vi "transfer char run_subvi_7_25_12a_JW.vi"(0 "VISA session":refnum<visa-resource-name>="GPIB0::17::INSTR", 5 "Var1 sweep settings":T4={"start"=40.0, "stop"=-40.0, "step (linear only)"=-1.0, "sweep spacing (linear: 0)"=0, "sweep mode"=FALSE, "compliance (V)"=100.0, "compliance (A)"=0.001} {"compliance (A)" format="%^.2e"; "compliance (V)" format="%.2f"; "sweep spacing (linear: 0)" items=["linear", "log 10", "log 25", "log 50"]; "step (linear only)" format="%.2f"; "stop" format="%.2f"; "start" format="%.2f"}, 7 "Var2 step settings":T3={"compliance (A)"=0.001, "compliance (V)"=100.0, "start"=-2.0, "total points"=2, "step"=-38.0} {"step" format="%.2f"; "start" format="%.2f"; "compliance (V)" format="%.2f"; "compliance (A)" format="%^.2e"}, 9 "integration time":u32(slide) scale=0.0..2.0, 11 "Input Path":path, 13 "Sample Properties:":T1 {"Date Created" format="%<%x>T"}) -> (1 "Trap Density-STS":dbl, 3 "Trap Density-VT":dbl, 4 "Mobility":dbl, 6 "graphic display":cluster{"trace":dbl[], "trace":dbl[]}(graph), 8 "On/Off Current":dbl, 10 "XY Graph":cluster{dbl[], "trace":dbl[]}[](graph), 12 "Vt":dbl, 14 "STS":dbl, 15 "error?":errorcluster)   [LabVIEW 2011]
uses:
  <vilib>/Utility/file.llb/Write To Spreadsheet File (DBL).vi
  <vilib>/Utility/file.llb/Read From Spreadsheet File (string).vi
  <vilib>/Utility/file.llb/Write To Spreadsheet File (string).vi
  <vilib>/Analysis/NI_AALPro.lvlib
panel:
  out "Array":string[][](array[string])
  in  "Output Path":path
  in  "Temp (K)":dbl=0.001 format="%^.2e"
  in  "NumPts":dbl=5.0
  out "Numeric":dbl
  out "Max R":i32[](listbox)
  out "min r":dbl
  out "max r":dbl
  out "error? 2":errorcluster
  in  "MAXIMUM":ext format="%.2e"
  in  "MINIMUM":ext=-1e-05 format="%_2e"
  out "graphic display 2":cluster{"trace":dbl[], "trace":dbl[]}(graph)
  in  "Y1 axis":string="Id"
  in  "Y2 axis settings":T2 {"MAXIMUM" format="%.9f"; "MINIMUM" format="%.9f"}
  in  "wait time parameter":dbl=1.0
  in  "Value (Either V or A) 4":dbl
  in  "Value (Either V or A) 3":dbl
  in  "Value (Either V or A) 2":dbl
  in  "Value (V or A)":dbl
  in  "compliance (A)":dbl=0.001 format="%^.2e"
  in  "compliance (V)":dbl=100.0 format="%^.2e"
  in  "Iname":string="Is"
  in  "Vname":string="Vs"
  in  "Function":u16(ring)=4 items=["disabled", "Var1", "Var2", "Var1'", "Constant"]
  in  "Mode":u16(ring)=4 items=["V", "I", "VPulse", "IPulse", "Common"]
  in  "Iname 4":string="I4"
  in  "Vname 4":string="V4"
  in  "Function 4":u16(ring)=4 items=["disabled", "Var1", "Var2", "Var1'", "Constant"]
  in  "Mode 4":u16(ring) items=["V", "I", "VPulse", "IPulse", "Common"]
  in  "Iname 3":string="Ig"
  in  "Vname 3":string="Vg"
  in  "Function 3":u16(ring)=1 items=["disabled", "Var1", "Var2", "Var1'", "Constant"]
  in  "Mode 3":u16(ring) items=["V", "I", "VPulse", "IPulse", "Common"]
  in  "Iname 2":string="Id"
  in  "Vname 2":string="Vd"
  in  "Function 2":u16(ring)=2 items=["disabled", "Var1", "Var2", "Var1'", "Constant"]
  in  "Mode 2":u16(ring) items=["V", "I", "VPulse", "IPulse", "Common"]
  in  "reset":bool=TRUE
  # "SMU1"
  # "SMU2"
  # "SMU3"
  # "SMU4"
  # "Sample Properties:"
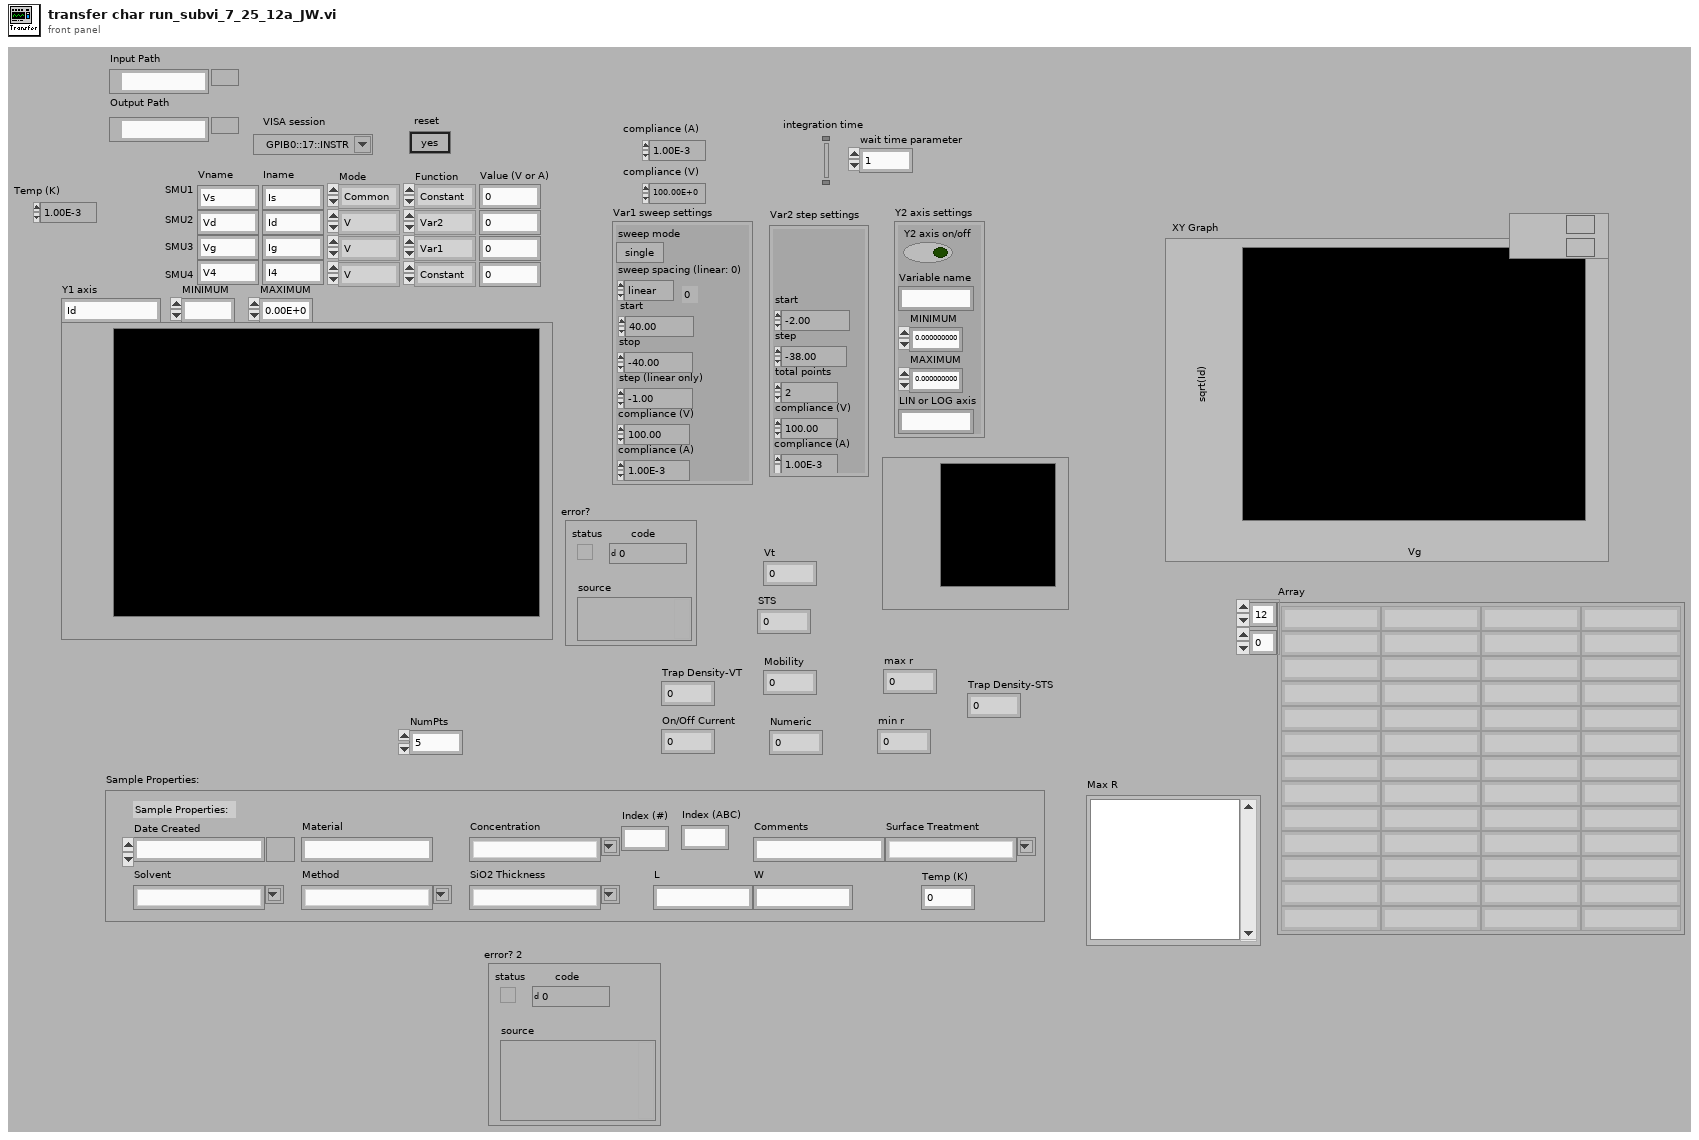
[diagram p1: front panel]
types:
  T1 = cluster{"Date Created":timestamp, "Material":string, "Solvent":string, "Concentration":string, "Method":string, "SiO2 Thickness":string, "Index (#)":string, "Index (ABC)":string, "L":string, "W":string, "Surface Treatment":string, "Comments":string, "Temp (K)":dbl}
  T2 = cluster{"Y2 axis on/off":bool, "MINIMUM":ext, "MAXIMUM":ext, "Variable name":string, "LIN or LOG axis":string}
  T3 = cluster{"compliance (A)":dbl, "compliance (V)":dbl, "start":dbl, "total points":u16, "step":dbl}
  T4 = cluster{"start":dbl, "stop":dbl, "step (linear only)":dbl, "sweep spacing (linear: 0)":u16, "sweep mode":bool, "compliance (V)":dbl, "compliance (A)":dbl}
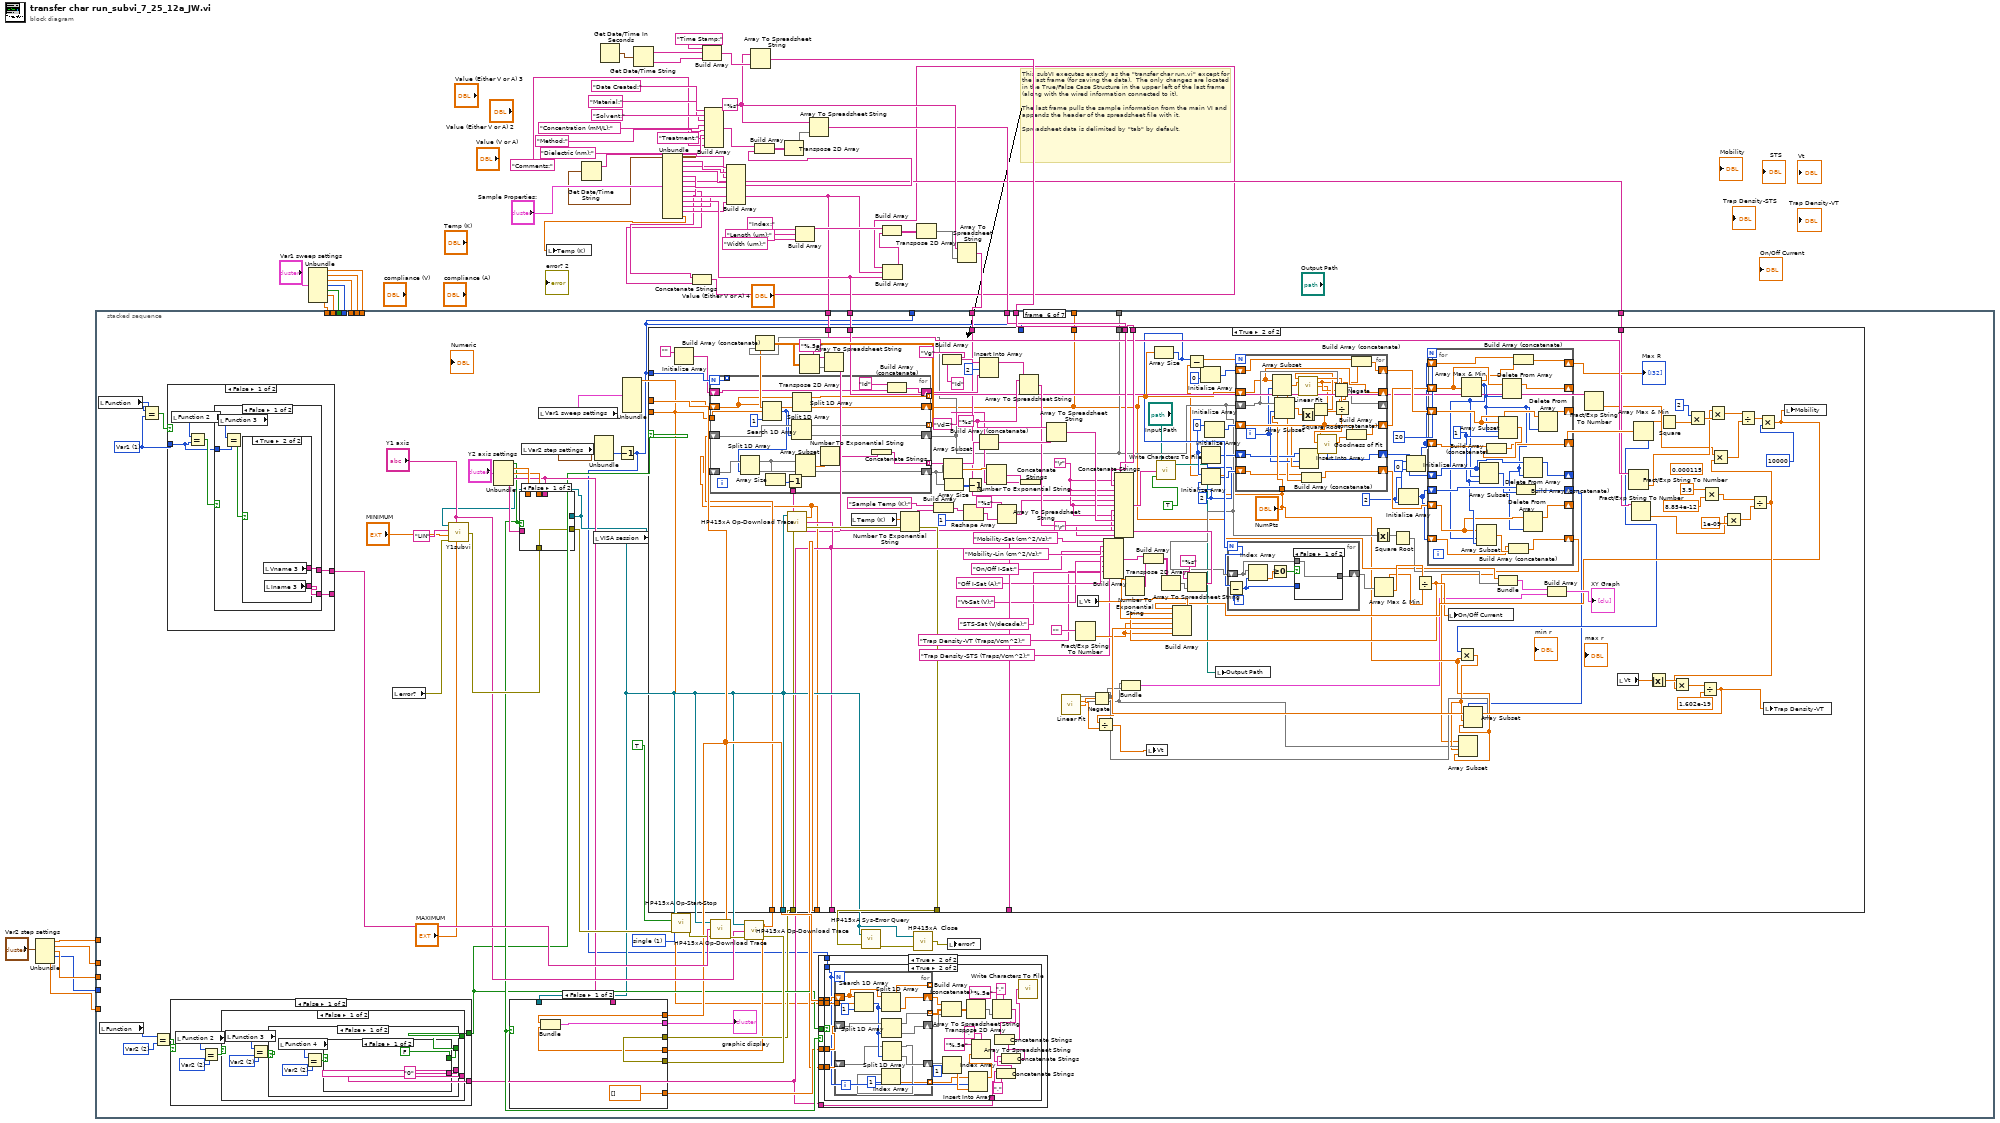
[diagram p0: block diagram]
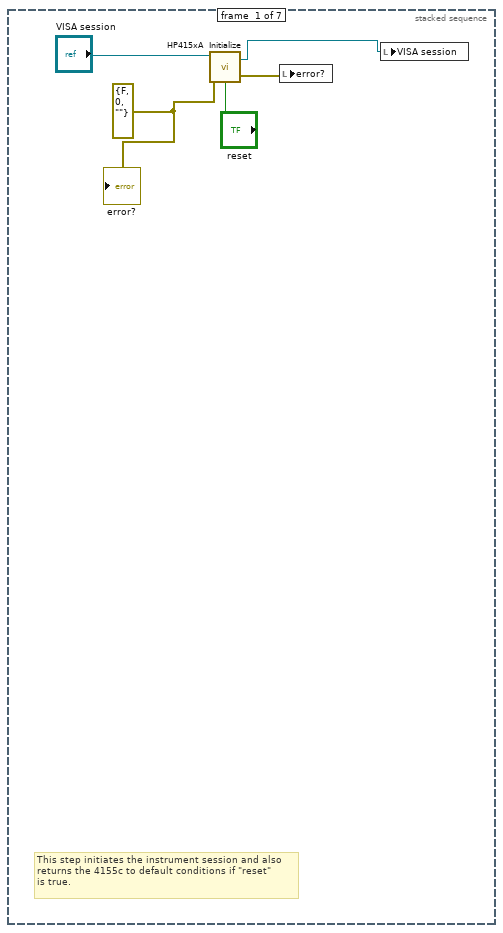
[diagram p2: hidden frame]
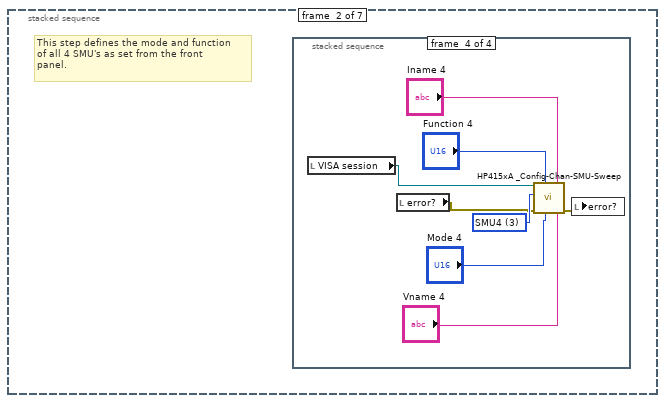
[diagram p3: hidden frame]
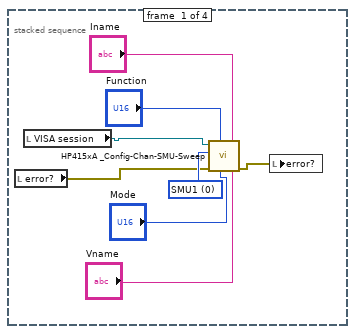
[diagram p4: hidden frame]
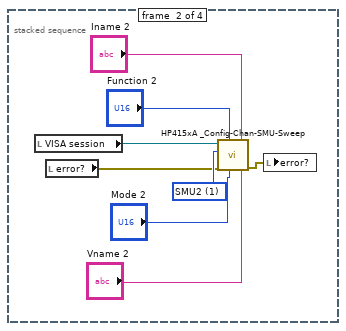
[diagram p5: hidden frame]
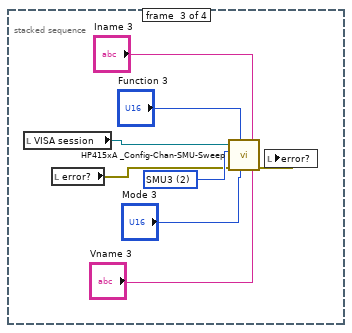
[diagram p6: hidden frame]
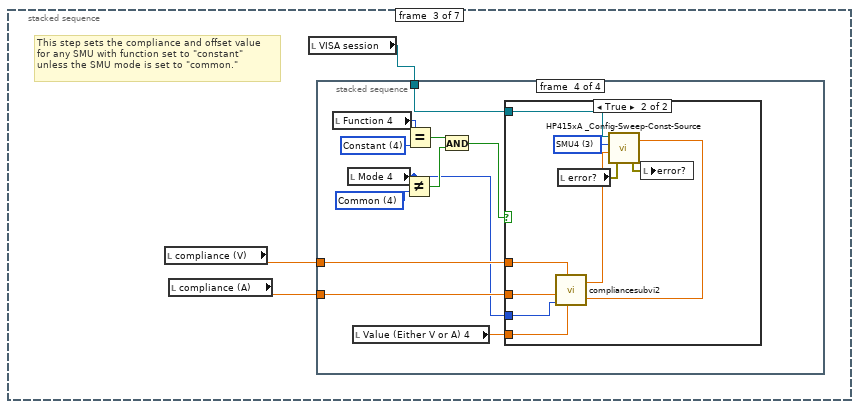
[diagram p7: hidden frame]
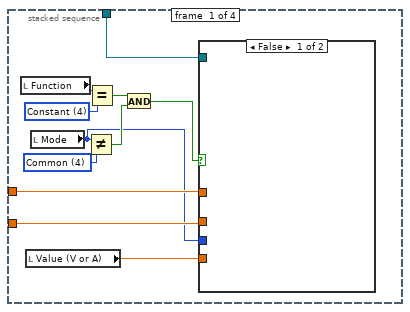
[diagram p8: hidden frame]
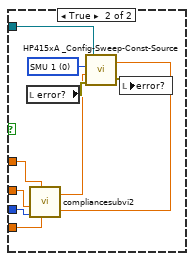
[diagram p9: hidden frame]
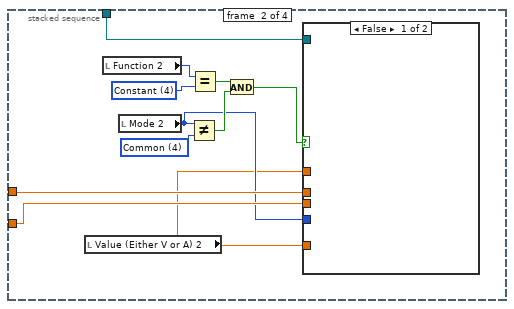
[diagram p10: hidden frame]
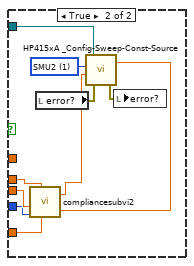
[diagram p11: hidden frame]
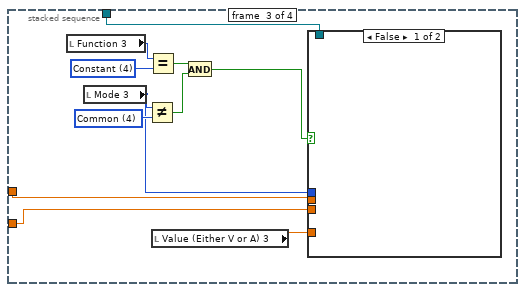
[diagram p12: hidden frame]
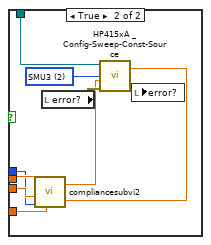
[diagram p13: hidden frame]
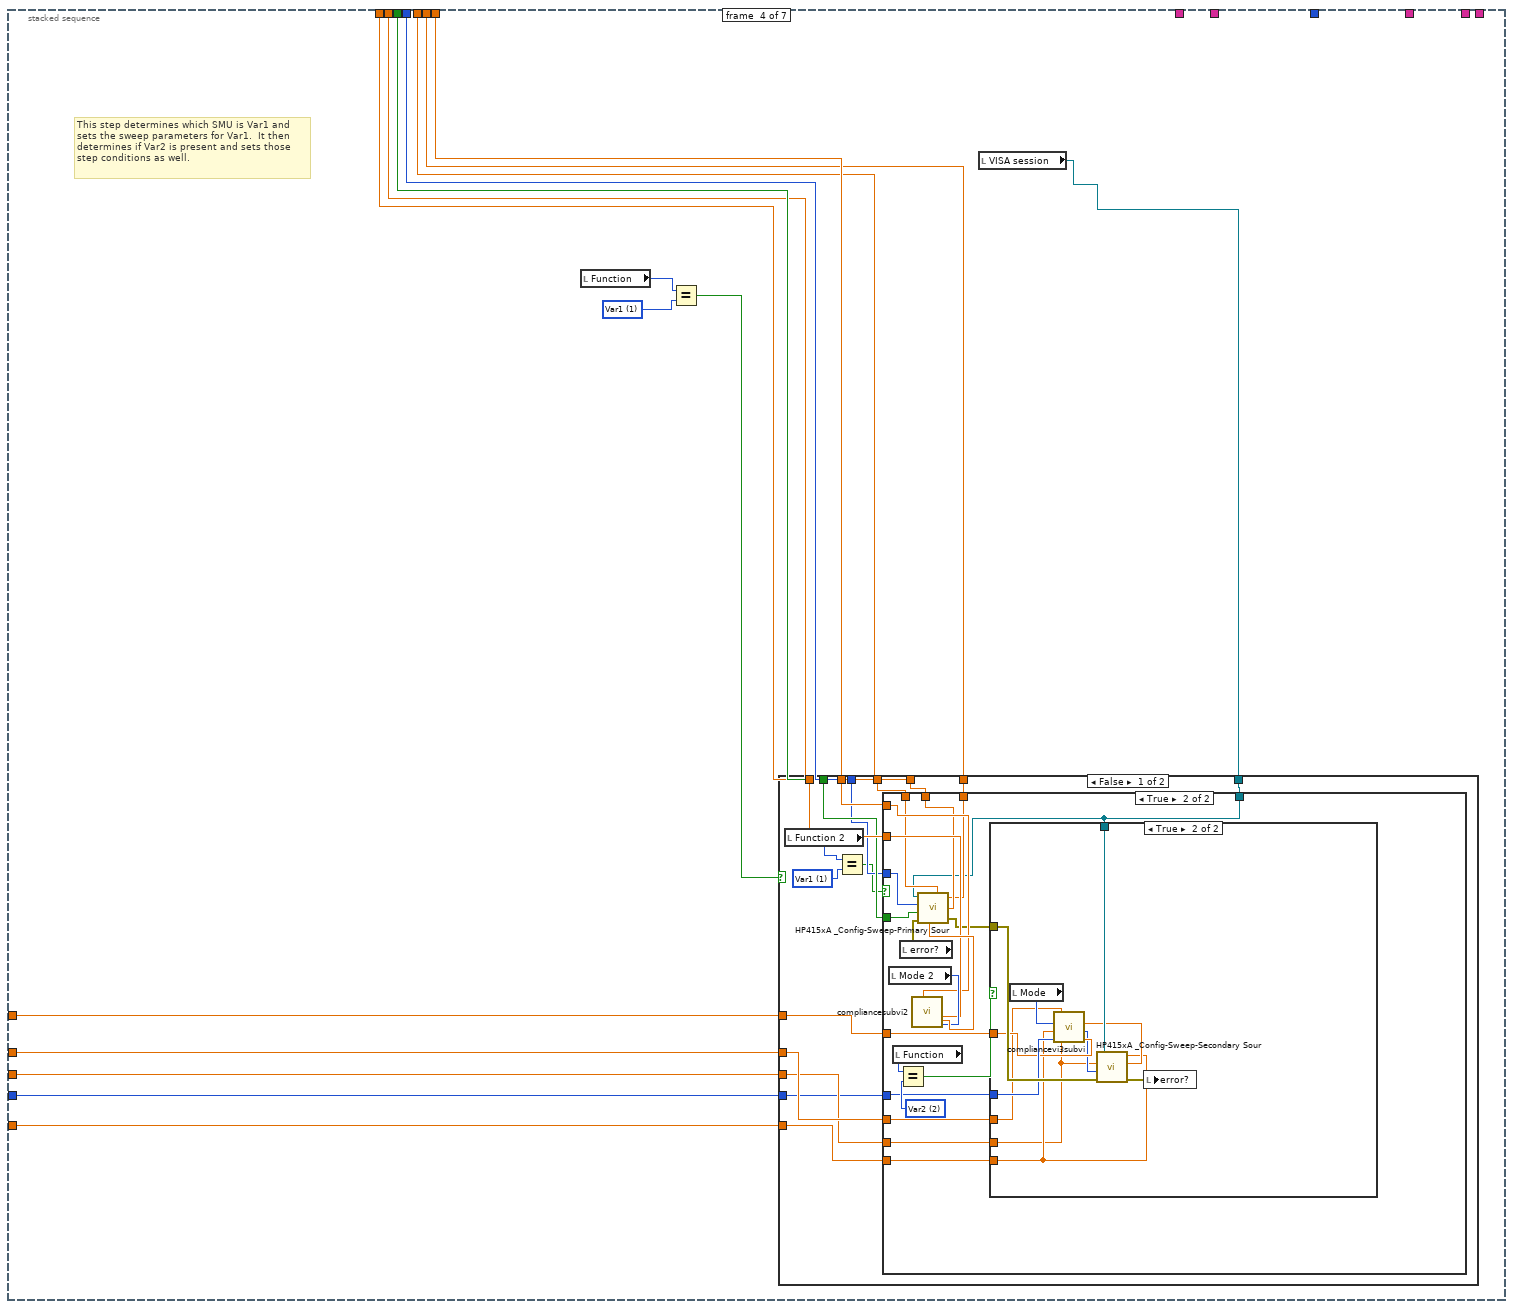
[diagram p15: hidden frame]
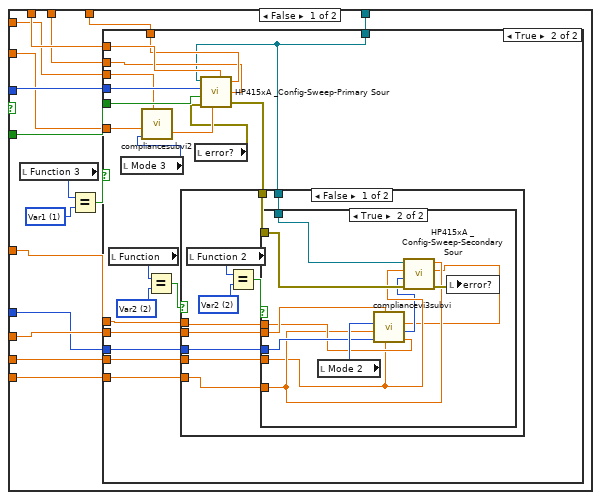
[diagram p16: hidden frame]
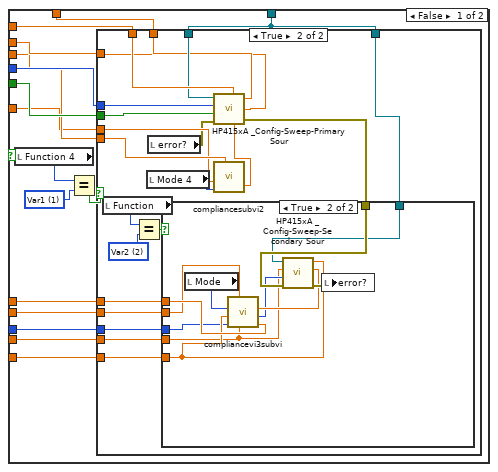
[diagram p17: hidden frame]
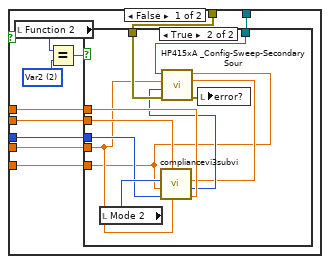
[diagram p19: hidden frame]
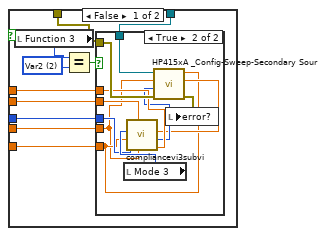
[diagram p20: hidden frame]
diagram:
  w31 = "%s"
  # "This subVI executes exactly as the \"transfer char run.vi\" except for the last frame (for saving the data).  The only changes are located in the True/False Case Structure in the upper left of the last frame (along with the wired information connected to it). \n\nThe last frame pulls the sample information from the main VI and appends the header of the spreadsheet file with it.\n\nSpreadsheet data is delimited by \"tab\" by default."
  n1 = Unbundle("Var2 step settings") -> ("compliance (A)"=w49:dbl, "compliance (V)"=w48:dbl, "start"=w47:dbl, "total points"=w46:u16, "step"=w45:dbl)
  n2 = Unbundle("Var1 sweep settings") -> ("start"=w57:dbl, "stop"=w56:dbl, "step (linear only)"=w55:dbl, "sweep spacing (linear: 0)"=w54:u16, "sweep mode"=w53:bool, "compliance (V)"=w52:dbl, "compliance (A)"=w51:dbl)
  n3 = Get Date/Time In Seconds() -> (seconds since 1Jan1904=w38:timestamp)
  n4 = Get Date/Time String(seconds (now)=w38) -> (date string=w37:string, time string=w36:string)  [unwired: 2 in]
  n5 = Unbundle("Sample Properties:") -> ("Date Created"=w16:timestamp, "Material"=w15:string, "Solvent"=w11:string, "Concentration"=w10:string, "Method"=w14:string, "SiO2 Thickness"=w9:string, "Index (#)"=w4:string, "Index (ABC)"=w3:string, "L"=w7:string, "W"=w8:string, "Surface Treatment"=w6:string, "Comments"=w5:string, "Temp (K)"=w1:dbl)
  n6 = local write "Temp (K)"(w1) -> ()
  n7 = Get Date/Time String(seconds (now)=w16) -> (date string=w43:string)  [unwired: 2 in, 1 out]
  n8 = Concatenate Strings(w4, w3) -> (w2:string)
  n9 = Build Array("Time Stamp:", w37, w36) -> (w35:string[])
  n10 = Build Array("Date Created:", "Material:", "Solvent:", "Concentration (mM/L):", "Method:", "Dielectric (nm):", "Treatment:", "Comments:") -> (w26:string[])
  n11 = Build Array(w43, w15, w11, w10, w14, w9, w6, w5) -> (w25:string[])
  n12 = Array To Spreadsheet String(array=w35, 3:w31) -> (spreadsheet string=w27:string)  [unwired: 1 in]
  n13 = Build Array(w26, w25) -> (w24:string[][])
  n14 = Transpose 2D Array(2D array=w24) -> (transposed array=w23:string[][])
  n15 = Build Array("Index:", "Length (um):", "Width (um):") -> (w22:string[])
  n16 = Array To Spreadsheet String(array=w23, 3:w31) -> (spreadsheet string=w30:string)  [unwired: 1 in]
  n17 = Build Array(w2, w7, w8) -> (w21:string[])
  n18 = Build Array(w22, w21) -> (w20:string[][])
  n19 = Transpose 2D Array(2D array=w20) -> (transposed array=w19:string[][])
  n20 = Array To Spreadsheet String(array=w19, 3:w31) -> (spreadsheet string=w18:string)  [unwired: 1 in]
  n21 = stacked-sequence {
    tunnel: w57 -> [_ _ _ w194 _ _ _]
    tunnel: w56 -> [_ _ _ w193 _ _ _]
    tunnel: w55 -> [_ _ _ w192 _ _ _]
    tunnel: w54 -> [_ _ _ w191 _ _ _]
    tunnel: w53 -> [_ _ _ w190 _ _ _]
    tunnel: w52 -> [_ _ _ w189 _ _ _]
    tunnel: w51 -> [_ _ _ w188 _ _ _]
    tunnel: w49 -> [_ _ _ w187 _ _ _]
    tunnel: w48 -> [_ _ _ w186 _ _ _]
    tunnel: w47 -> [_ _ _ w185 _ _ _]
    tunnel: w46 -> [_ _ _ w184 _ _ _]
    tunnel: w45 -> [_ _ _ w183 _ _ _]
    tunnel: w27 -> [_ _ _ _ _ w557 _]
    tunnel: w30 -> [_ _ _ _ _ w556 _]
    tunnel: w18 -> [_ _ _ _ _ w555 _]
    tunnel: [_ _ _ _ _ w554 _] -> _
    tunnel: [_ _ _ _ _ w553 _] -> _
    tunnel: [_ _ _ _ _ w550 _] -> _
    tunnel: w8 -> [_ _ _ _ _ w552 _]
    tunnel: w7 -> [_ _ _ _ _ w551 _]
    tunnel: w9 -> [_ _ _ _ _ w549 _]
    frame #0 {
      w62 = errorcluster {"status"=FALSE, "code"=0, "source"=""} ("error out")
      # "This step initiates the instrument session and also\nreturns the 4155c to default conditions if \"reset\"\nis true."
      n22 = call "HP415xA  Initialize.vi"("instrument descriptor"="VISA session", "reset"="reset", "error in (no error)"=w62) -> ("VISA session"=w59:refnum<visa-resource-name>, "error out"=w61:errorcluster)  [unwired: 2 in]
      n23 = local write "error?"(w61) -> ()
      n24 = local write "VISA session"(w59) -> ()
      "error?" <- w62
    }
    frame #1 {
      # "This step defines the mode and function\nof all 4 SMU's as set from the front\npanel."
      n25 = stacked-sequence {
        frame #0 {
          w71 = u32 0 items=["SMU1  ", "SMU2  ", "SMU3  ", "SMU4  ", "SMU5  ", "SMU6  "] ("unit to configure")
          n26 = local read "error?"() -> (w66:errorcluster)
          n27 = local read "VISA session"() -> (w64:refnum<visa-resource-name>)
          n28 = call "HP415xA _Config-Chan-SMU-Sweep.vi"("V name (max 6 chars)"="Vname", "I name (max 6 chars)"="Iname", "mode"="Mode", "function"="Function", "error in (no error)"=w66, "unit to configure"=w71, "VISA session"=w64) -> ("error out"=w65:errorcluster)  [unwired: 2 in]
          n29 = local write "error?"(w65) -> ()
        }
        frame #1 {
          w75 = u32 1 items=["SMU1  ", "SMU2  ", "SMU3  ", "SMU4  ", "SMU5  ", "SMU6  "] ("unit to configure")
          n30 = local read "VISA session"() -> (w72:refnum<visa-resource-name>)
          n31 = local read "error?"() -> (w73:errorcluster)
          n32 = call "HP415xA _Config-Chan-SMU-Sweep.vi"("V name (max 6 chars)"="Vname 2", "I name (max 6 chars)"="Iname 2", "mode"="Mode 2", "function"="Function 2", "error in (no error)"=w73, "unit to configure"=w75, "VISA session"=w72) -> ("error out"=w74:errorcluster)  [unwired: 2 in]
          n33 = local write "error?"(w74) -> ()
        }
        frame #2 {
          w83 = u32 2 items=["SMU1  ", "SMU2  ", "SMU3  ", "SMU4  ", "SMU5  ", "SMU6  "] ("unit to configure")
          n34 = local read "VISA session"() -> (w80:refnum<visa-resource-name>)
          n35 = local read "error?"() -> (w81:errorcluster)
          n36 = call "HP415xA _Config-Chan-SMU-Sweep.vi"("V name (max 6 chars)"="Vname 3", "I name (max 6 chars)"="Iname 3", "mode"="Mode 3", "function"="Function 3", "error in (no error)"=w81, "unit to configure"=w83, "VISA session"=w80) -> ("error out"=w82:errorcluster)  [unwired: 2 in]
          n37 = local write "error?"(w82) -> ()
        }
        frame #3 {
          w91 = u32 3 items=["SMU1  ", "SMU2  ", "SMU3  ", "SMU4  ", "SMU5  ", "SMU6  "] ("unit to configure")
          n38 = local read "VISA session"() -> (w88:refnum<visa-resource-name>)
          n39 = local read "error?"() -> (w90:errorcluster)
          n40 = call "HP415xA _Config-Chan-SMU-Sweep.vi"("V name (max 6 chars)"="Vname 4", "I name (max 6 chars)"="Iname 4", "mode"="Mode 4", "function"="Function 4", "error in (no error)"=w90, "unit to configure"=w91, "VISA session"=w88) -> ("error out"=w89:errorcluster)  [unwired: 2 in]
          n41 = local write "error?"(w89) -> ()
        }
      }
    }
    frame #2 {
      # "This step sets the compliance and offset value\nfor any SMU with function set to \"constant\"\nunless the SMU mode is set to \"common.\""
      n42 = local read "compliance (V)"() -> (w97:dbl)
      n43 = local read "compliance (A)"() -> (w98:dbl)
      n44 = local read "VISA session"() -> (w96:refnum<visa-resource-name>)
      n45 = stacked-sequence {
        tunnel: w96 -> [w107 w127 w146 w166]
        tunnel: w98 -> [w101 w123 w144 w164]
        tunnel: w97 -> [w100 w122 w143 w165]
        frame #0 {
          w105 = u16 4 items=["V", "I", "VPulse", "IPulse", "Common"] ("Mode")
          w109 = u16 4 items=["disabled", "Var1", "Var2", "Var1'", "Constant"] ("Function")
          n46 = local read "Function"() -> (w108:u16)
          n47 = local read "Value (V or A)"() -> (w102:dbl)
          n48 = local read "Mode"() -> (w99:u16)
          n49 = Not Equal?(x=w99, y=w105) -> (x != y?=w104:bool)
          n50 = Equal?(x=w108, y=w109) -> (x = y?=w106:bool)
          n51 = And(x=w106, y=w104) -> (x .and. y?=w103:bool)
          n52 = case shown="False" w103 {
            tunnel: w107 -> [_ w119]
            tunnel: w100 -> [_ w115]
            tunnel: w101 -> [_ w114]
            tunnel: w102 -> [_ w111]
            tunnel: w99 -> [_ w112]
            frame False {
            }
            frame True {
              w118 = u16 0 items=["SMU 1", "SMU2", "SMU3", "SMU4", "SMU5", "SMU6", "VSU1", "VSU2"] ("unit (SMU1:0)")
              n53 = local read "error?"() -> (w117:errorcluster)
              n54 = call "compliancesubvi2.vi"("Value1"=w111, "compliance (V)"=w115, "Mode"=w112, "compliance (A)"=w114) -> ("compliance"=w113:dbl, "constant"=w110:dbl)  [unwired: 2 in]
              n55 = call "HP415xA _Config-Sweep-Const-Source.vi"("compliance (SMUs only)"=w113, "error in (no error)"=w117, "source (V or A)"=w110, "unit (SMU1:0)"=w118, "VISA session"=w119) -> ("error out"=w116:errorcluster)
              n56 = local write "error?"(w116) -> ()
            }
          }
        }
        frame #1 {
          w124 = u16 4 items=["V", "I", "VPulse", "IPulse", "Common"] ("Mode 2")
          w125 = u16 4 items=["disabled", "Var1", "Var2", "Var1'", "Constant"] ("Function 2")
          n57 = local read "Value (Either V or A) 2"() -> (w120:dbl)
          n58 = local read "Function 2"() -> (w126:u16)
          n59 = local read "Mode 2"() -> (w121:u16)
          n60 = Not Equal?(x=w121, y=w124) -> (x != y?=w129:bool)
          n61 = Equal?(x=w126, y=w125) -> (x = y?=w130:bool)
          n62 = And(x=w130, y=w129) -> (x .and. y?=w128:bool)
          n63 = case shown="False" w128 {
            tunnel: w127 -> [_ w140]
            tunnel: w122 -> [_ w138]
            tunnel: w123 -> [_ w137]
            tunnel: w120 -> [_ _]
            tunnel: w121 -> [_ w133]
            tunnel: w120 -> [_ w132]
            frame False {
            }
            frame True {
              w139 = u16 1 items=["SMU 1", "SMU2", "SMU3", "SMU4", "SMU5", "SMU6", "VSU1", "VSU2"] ("unit (SMU1:0)")
              n64 = call "compliancesubvi2.vi"("Value1"=w132, "compliance (V)"=w138, "Mode"=w133, "compliance (A)"=w137) -> ("compliance"=w136:dbl, "constant"=w131:dbl)  [unwired: 2 in]
              n65 = local read "error?"() -> (w135:errorcluster)
              n66 = call "HP415xA _Config-Sweep-Const-Source.vi"("compliance (SMUs only)"=w136, "error in (no error)"=w135, "source (V or A)"=w131, "unit (SMU1:0)"=w139, "VISA session"=w140) -> ("error out"=w134:errorcluster)
              n67 = local write "error?"(w134) -> ()
            }
          }
        }
        frame #2 {
          w148 = u16 4 items=["V", "I", "VPulse", "IPulse", "Common"] ("Mode 2")
          w149 = u16 4 items=["disabled", "Var1", "Var2", "Var1'", "Constant"] ("Function 2")
          n68 = local read "Function 3"() -> (w147:u16)
          n69 = local read "Mode 3"() -> (w142:u16)
          n70 = Not Equal?(x=w142, y=w148) -> (x != y?=w150:bool)
          n71 = Equal?(x=w147, y=w149) -> (x = y?=w151:bool)
          n72 = local read "Value (Either V or A) 3"() -> (w145:dbl)
          n73 = And(x=w151, y=w150) -> (x .and. y?=w141:bool)
          n74 = case shown="False" w141 {
            tunnel: w146 -> [_ w159]
            tunnel: w145 -> [_ w153]
            tunnel: w144 -> [_ w156]
            tunnel: w143 -> [_ w155]
            tunnel: w142 -> [_ w154]
            frame False {
            }
            frame True {
              w158 = u16 2 items=["SMU 1", "SMU2", "SMU3", "SMU4", "SMU5", "SMU6", "VSU1", "VSU2"] ("unit (SMU1:0)")
              n75 = call "compliancesubvi2.vi"("Value1"=w153, "compliance (V)"=w155, "Mode"=w154, "compliance (A)"=w156) -> ("compliance"=w157:dbl, "constant"=w152:dbl)  [unwired: 2 in]
              n76 = local read "error?"() -> (w161:errorcluster)
              n77 = call "HP415xA _Config-Sweep-Const-Source.vi"("compliance (SMUs only)"=w157, "error in (no error)"=w161, "source (V or A)"=w152, "unit (SMU1:0)"=w158, "VISA session"=w159) -> ("error out"=w160:errorcluster)
              n78 = local write "error?"(w160) -> ()
            }
          }
        }
        frame #3 {
          w168 = u16 4 items=["V", "I", "VPulse", "IPulse", "Common"] ("Mode 4")
          w169 = u16 4 items=["disabled", "Var1", "Var2", "Var1'", "Constant"] ("Function 4")
          n79 = local read "Function 4"() -> (w170:u16)
          n80 = local read "Mode 4"() -> (w163:u16)
          n81 = local read "Value (Either V or A) 4"() -> (w162:dbl)
          n82 = Not Equal?(x=w163, y=w168) -> (x != y?=w171:bool)
          n83 = Equal?(x=w170, y=w169) -> (x = y?=w172:bool)
          n84 = And(x=w172, y=w171) -> (x .and. y?=w167:bool)
          n85 = case shown="True" w167 {
            tunnel: w166 -> [_ w181]
            tunnel: w165 -> [_ w177]
            tunnel: w164 -> [_ w178]
            tunnel: w163 -> [_ w176]
            tunnel: w162 -> [_ w175]
            frame False {
            }
            frame True {
              w182 = u16 3 items=["SMU 1", "SMU2", "SMU3", "SMU4", "SMU5", "SMU6", "VSU1", "VSU2"] ("unit (SMU1:0)")
              n86 = call "compliancesubvi2.vi"("Value1"=w175, "compliance (V)"=w177, "Mode"=w176, "compliance (A)"=w178) -> ("compliance"=w174:dbl, "constant"=w173:dbl)  [unwired: 2 in]
              n87 = local read "error?"() -> (w180:errorcluster)
              n88 = call "HP415xA _Config-Sweep-Const-Source.vi"("compliance (SMUs only)"=w174, "error in (no error)"=w180, "source (V or A)"=w173, "unit (SMU1:0)"=w182, "VISA session"=w181) -> ("error out"=w179:errorcluster)
              n89 = local write "error?"(w179) -> ()
            }
          }
        }
      }
    }
    frame #3 {
      w198 = u16 1 items=["disabled", "Var1", "Var2", "Var1'", "Constant"] ("Function")
      # "This step determines which SMU is Var1 and\nsets the sweep parameters for Var1.  It then\ndetermines if Var2 is present and sets those\nstep conditions as well."
      n90 = local read "Function"() -> (w197:u16)
      n91 = Equal?(x=w197, y=w198) -> (x = y?=w196:bool)
      n92 = local read "VISA session"() -> (w195:refnum<visa-resource-name>)
      n93 = case shown="False" w196 {
        tunnel: w189 -> [w211 w487]
        tunnel: w188 -> [w212 w486]
        tunnel: w191 -> [w209 w485]
        tunnel: w190 -> [w210 w484]
        tunnel: w192 -> [w206 w483]
        tunnel: w193 -> [w205 w482]
        tunnel: w194 -> [w207 w481]
        tunnel: w195 -> [w208 w470]
        tunnel: w187 -> [w203 w476]
        tunnel: w186 -> [w202 w475]
        tunnel: w185 -> [w201 w474]
        tunnel: w184 -> [w200 w473]
        tunnel: w183 -> [w199 w472]
        frame False {
          w214 = u16 1 items=["disabled", "Var1", "Var2", "Var1'", "Constant"] ("Function")
          n94 = local read "Function 2"() -> (w213:u16)
          n95 = Equal?(x=w213, y=w214) -> (x = y?=w204:bool)
          n96 = case shown="True" w204 {
            tunnel: w212 -> [w220 w413]
            tunnel: w211 -> [w221 w412]
            tunnel: w210 -> [w222 w411]
            tunnel: w209 -> [w223 w410]
            tunnel: w208 -> [w227 w399]
            tunnel: w207 -> [w226 w409]
            tunnel: w206 -> [w224 w408]
            tunnel: w205 -> [w225 w407]
            tunnel: w203 -> [w219 w402]
            tunnel: w202 -> [w218 w401]
            tunnel: w201 -> [w216 w400]
            tunnel: w200 -> [w217 w397]
            tunnel: w199 -> [w215 w396]
            frame False {
              w230 = u16 1 items=["disabled", "Var1", "Var2", "Var1'", "Constant"] ("Function")
              n97 = local read "Function 3"() -> (w229:u16)
              n98 = Equal?(x=w229, y=w230) -> (x = y?=w228:bool)
              n99 = case shown="True" w228 {
                tunnel: w227 -> [w231 w324]
                tunnel: w226 -> [w243 w341]
                tunnel: w225 -> [w240 w340]
                tunnel: w224 -> [w239 w339]
                tunnel: w223 -> [w242 w338]
                tunnel: w222 -> [w241 w337]
                tunnel: w221 -> [w238 w336]
                tunnel: w220 -> [w237 w335]
                tunnel: w219 -> [w236 w328]
                tunnel: w218 -> [w235 w327]
                tunnel: w217 -> [w234 w326]
                tunnel: w216 -> [w233 w323]
                tunnel: w215 -> [w232 w322]
                frame False {
                  w246 = u16 1 items=["disabled", "Var1", "Var2", "Var1'", "Constant"] ("Function")
                  n100 = local read "Function 4"() -> (w245:u16)
                  n101 = Equal?(x=w245, y=w246) -> (x = y?=w244:bool)
                  n102 = case shown="True" w244 {
                    tunnel: w243 -> [_ w265]
                    tunnel: w231 -> [_ w264]
                    tunnel: w242 -> [_ w263]
                    tunnel: w241 -> [_ w262]
                    tunnel: w240 -> [_ w261]
                    tunnel: w239 -> [_ w260]
                    tunnel: w238 -> [_ w259]
                    tunnel: w237 -> [_ w258]
                    tunnel: w236 -> [_ w253]
                    tunnel: w235 -> [_ w252]
                    tunnel: w234 -> [_ w251]
                    tunnel: w233 -> [_ w250]
                    tunnel: w232 -> [_ w249]
                    tunnel: w231 -> [_ w247]
                    frame False {
                    }
                    frame True {
                      w256 = u16 2 items=["disabled", "Var1", "Var2", "Var1'", "Constant"] ("Function")
                      n103 = local read "Function"() -> (w255:u16)
                      n104 = Equal?(x=w255, y=w256) -> (x = y?=w254:bool)
                      n105 = local read "Mode 4"() -> (w267:u16)
                      n106 = local read "error?"() -> (w257:errorcluster)
                      n107 = call "compliancesubvi2.vi"("compliance (V)"=w259, "Mode"=w267, "compliance (A)"=w258) -> ("compliance"=w266:dbl)  [unwired: 3 in, 1 out]
                      n108 = call "HP415xA _Config-Sweep-Primary Sour.vi"("step (linear only)"=w260, "stop"=w261, "start"=w265, "compliance"=w266, "error in (no error)"=w257, "sweep mode"=w262, "sweep spacing (linear: 0)"=w263, "VISA session"=w264) -> ("error out"=w248:errorcluster)  [unwired: 2 in]
                      n109 = case shown="True" w254 {
                        tunnel: w253 -> [w274 w317]
                        tunnel: w252 -> [w273 w312]
                        tunnel: w251 -> [w272 w311]
                        tunnel: w250 -> [w271 w313]
                        tunnel: w249 -> [w270 w316]
                        tunnel: w248 -> [w269 w319]
                        tunnel: w247 -> [w268 w318]
                        frame False {
                          w277 = u16 2 items=["disabled", "Var1", "Var2", "Var1'", "Constant"] ("Function")
                          n110 = local read "Function 2"() -> (w276:u16)
                          n111 = Equal?(x=w276, y=w277) -> (x = y?=w275:bool)
                          n112 = case shown="True" w275 {
                            tunnel: w274 -> [w285 w305]
                            tunnel: w273 -> [w284 w306]
                            tunnel: w272 -> [w283 w304]
                            tunnel: w271 -> [w282 w302]
                            tunnel: w270 -> [w281 w300]
                            tunnel: w269 -> [w280 w310]
                            tunnel: w268 -> [w278 w309]
                            frame False {
                              w287 = u16 2 items=["disabled", "Var1", "Var2", "Var1'", "Constant"] ("Function")
                              n113 = local read "Function 3"() -> (w279:u16)
                              n114 = Equal?(x=w279, y=w287) -> (x = y?=w286:bool)
                              n115 = case shown="True" w286 {
                                tunnel: w285 -> [_ w293]
                                tunnel: w284 -> [_ w294]
                                tunnel: w283 -> [_ w295]
                                tunnel: w282 -> [_ w289]
                                tunnel: w281 -> [_ w290]
                                tunnel: w280 -> [w288 w299]
                                tunnel: w278 -> [_ w298]
                                frame False {
                                n116 = local write "error?"(w288) -> ()
                                }
                                frame True {
                                n117 = local read "Mode 3"() -> (w297:u16)
                                n118 = call "compliancevi3subvi.vi"("compliance (A)"=w293, "start"=w289, "compliance (V)"=w294, "total points"=w295, "step"=w290, "Mode"=w297) -> ("total points 2"=w292:u16, "compliance"=w291:dbl)  [unwired: 1 in, 1 out]
                                n119 = call "HP415xA _Config-Sweep-Secondary Sour.vi"("compliance"=w291, "step"=w290, "error in (no error)"=w299, "total points"=w292, "start"=w289, "VISA session"=w298) -> ("error out"=w296:errorcluster)  [unwired: 1 in]
                                n120 = local write "error?"(w296) -> ()
                                }
                              }
                            }
                            frame True {
                              n121 = local read "Mode 2"() -> (w308:u16)
                              n122 = call "compliancevi3subvi.vi"("compliance (A)"=w305, "start"=w302, "compliance (V)"=w306, "total points"=w304, "step"=w300, "Mode"=w308) -> ("total points 2"=w303:u16, "compliance"=w301:dbl)  [unwired: 1 in, 1 out]
                              n123 = call "HP415xA _Config-Sweep-Secondary Sour.vi"("compliance"=w301, "step"=w300, "error in (no error)"=w310, "total points"=w303, "start"=w302, "VISA session"=w309) -> ("error out"=w307:errorcluster)  [unwired: 1 in]
                              n124 = local write "error?"(w307) -> ()
                            }
                          }
                        }
                        frame True {
                          n125 = local read "Mode"() -> (w321:u16)
                          n126 = call "compliancevi3subvi.vi"("compliance (A)"=w317, "start"=w313, "compliance (V)"=w312, "total points"=w311, "step"=w316, "Mode"=w321) -> ("total points 2"=w314:u16, "compliance"=w315:dbl)  [unwired: 1 in, 1 out]
                          n127 = call "HP415xA _Config-Sweep-Secondary Sour.vi"("compliance"=w315, "step"=w316, "error in (no error)"=w319, "total points"=w314, "start"=w313, "VISA session"=w318) -> ("error out"=w320:errorcluster)  [unwired: 1 in]
                          n128 = local write "error?"(w320) -> ()
                        }
                      }
                    }
                  }
                }
                frame True {
                  w331 = u16 2 items=["disabled", "Var1", "Var2", "Var1'", "Constant"] ("Function")
                  n129 = local read "Function"() -> (w330:u16)
                  n130 = local read "Mode 3"() -> (w333:u16)
                  n131 = call "compliancesubvi2.vi"("compliance (V)"=w336, "Mode"=w333, "compliance (A)"=w335) -> ("compliance"=w334:dbl)  [unwired: 3 in, 1 out]
                  n132 = Equal?(x=w330, y=w331) -> (x = y?=w329:bool)
                  n133 = local read "error?"() -> (w332:errorcluster)
                  n134 = call "HP415xA _Config-Sweep-Primary Sour.vi"("step (linear only)"=w339, "stop"=w340, "start"=w341, "compliance"=w334, "error in (no error)"=w332, "sweep mode"=w337, "sweep spacing (linear: 0)"=w338, "VISA session"=w324) -> ("error out"=w325:errorcluster)  [unwired: 2 in]
                  n135 = case shown="False" w329 {
                    tunnel: w328 -> [w346 w391]
                    tunnel: w327 -> [w345 w390]
                    tunnel: w326 -> [w343 w389]
                    tunnel: w325 -> [w348 w394]
                    tunnel: w324 -> [w347 w393]
                    tunnel: w323 -> [w342 w386]
                    tunnel: w322 -> [w344 w385]
                    frame False {
                      w351 = u16 2 items=["disabled", "Var1", "Var2", "Var1'", "Constant"] ("Function")
                      n136 = local read "Function 2"() -> (w350:u16)
                      n137 = Equal?(x=w350, y=w351) -> (x = y?=w349:bool)
                      n138 = case shown="True" w349 {
                        tunnel: w348 -> [w358 w383]
                        tunnel: w347 -> [w357 w382]
                        tunnel: w346 -> [w356 w378]
                        tunnel: w345 -> [w355 w379]
                        tunnel: w344 -> [w352 w377]
                        tunnel: w343 -> [w354 w380]
                        tunnel: w342 -> [w353 w376]
                        frame False {
                          w361 = u16 2 items=["disabled", "Var1", "Var2", "Var1'", "Constant"] ("Function")
                          n139 = local read "Function 4"() -> (w360:u16)
                          n140 = Equal?(x=w360, y=w361) -> (x = y?=w359:bool)
                          n141 = case shown="True" w359 {
                            tunnel: w358 -> [w362 w371]
                            tunnel: w357 -> [_ w372]
                            tunnel: w356 -> [_ w368]
                            tunnel: w355 -> [_ w369]
                            tunnel: w354 -> [_ w367]
                            tunnel: w353 -> [_ w364]
                            tunnel: w352 -> [_ w363]
                            frame False {
                              n142 = local write "error?"(w362) -> ()
                            }
                            frame True {
                              n143 = local read "Mode 4"() -> (w373:u16)
                              n144 = call "compliancevi3subvi.vi"("compliance (A)"=w368, "start"=w364, "compliance (V)"=w369, "total points"=w367, "step"=w363, "Mode"=w373) -> ("total points 2"=w366:u16, "compliance"=w365:dbl)  [unwired: 1 in, 1 out]
                              n145 = call "HP415xA _Config-Sweep-Secondary Sour.vi"("compliance"=w365, "step"=w363, "error in (no error)"=w371, "total points"=w366, "start"=w364, "VISA session"=w372) -> ("error out"=w370:errorcluster)  [unwired: 1 in]
                              n146 = local write "error?"(w370) -> ()
                            }
                          }
                        }
                        frame True {
                          n147 = local read "Mode 2"() -> (w384:u16)
                          n148 = call "compliancevi3subvi.vi"("compliance (A)"=w378, "start"=w376, "compliance (V)"=w379, "total points"=w380, "step"=w377, "Mode"=w384) -> ("total points 2"=w375:u16, "compliance"=w374:dbl)  [unwired: 1 in, 1 out]
                          n149 = call "HP415xA _Config-Sweep-Secondary Sour.vi"("compliance"=w374, "step"=w377, "error in (no error)"=w383, "total points"=w375, "start"=w376, "VISA session"=w382) -> ("error out"=w381:errorcluster)  [unwired: 1 in]
                          n150 = local write "error?"(w381) -> ()
                        }
                      }
                    }
                    frame True {
                      n151 = local read "Mode"() -> (w395:u16)
                      n152 = call "compliancevi3subvi.vi"("compliance (A)"=w391, "start"=w386, "compliance (V)"=w390, "total points"=w389, "step"=w385, "Mode"=w395) -> ("total points 2"=w388:u16, "compliance"=w387:dbl)  [unwired: 1 in, 1 out]
                      n153 = call "HP415xA _Config-Sweep-Secondary Sour.vi"("compliance"=w387, "step"=w385, "error in (no error)"=w394, "total points"=w388, "start"=w386, "VISA session"=w393) -> ("error out"=w392:errorcluster)  [unwired: 1 in]
                      n154 = local write "error?"(w392) -> ()
                    }
                  }
                }
              }
            }
            frame True {
              w405 = u16 2 items=["disabled", "Var1", "Var2", "Var1'", "Constant"] ("Function")
              n155 = local read "Mode 2"() -> (w414:u16)
              n156 = local read "Function"() -> (w404:u16)
              n157 = Equal?(x=w404, y=w405) -> (x = y?=w403:bool)
              n158 = local read "error?"() -> (w406:errorcluster)
              n159 = call "compliancesubvi2.vi"("compliance (V)"=w412, "Mode"=w414, "compliance (A)"=w413) -> ("compliance"=w415:dbl)  [unwired: 3 in, 1 out]
              n160 = call "HP415xA _Config-Sweep-Primary Sour.vi"("step (linear only)"=w408, "stop"=w407, "start"=w409, "compliance"=w415, "error in (no error)"=w406, "sweep mode"=w411, "sweep spacing (linear: 0)"=w410, "VISA session"=w399) -> ("error out"=w398:errorcluster)  [unwired: 2 in]
              n161 = case shown="True" w403 {
                tunnel: w402 -> [w421 w464]
                tunnel: w401 -> [w420 w463]
                tunnel: w400 -> [w418 w459]
                tunnel: w399 -> [w423 w469]
                tunnel: w398 -> [w417 w468]
                tunnel: w397 -> [w419 w465]
                tunnel: w396 -> [w416 w461]
                frame False {
                  w425 = u16 2 items=["disabled", "Var1", "Var2", "Var1'", "Constant"] ("Function")
                  n162 = local read "Function 3"() -> (w424:u16)
                  n163 = Equal?(x=w424, y=w425) -> (x = y?=w422:bool)
                  n164 = case shown="True" w422 {
                    tunnel: w423 -> [w431 w457]
                    tunnel: w421 -> [w430 w454]
                    tunnel: w420 -> [w428 w452]
                    tunnel: w419 -> [w429 w453]
                    tunnel: w418 -> [w426 w450]
                    tunnel: w417 -> [w432 w456]
                    tunnel: w416 -> [w427 w448]
                    frame False {
                      w435 = u16 2 items=["disabled", "Var1", "Var2", "Var1'", "Constant"] ("Function")
                      n165 = local read "Function 4"() -> (w434:u16)
                      n166 = Equal?(x=w434, y=w435) -> (x = y?=w433:bool)
                      n167 = case shown="True" w433 {
                        tunnel: w432 -> [w436 w447]
                        tunnel: w431 -> [_ w446]
                        tunnel: w430 -> [_ w443]
                        tunnel: w429 -> [_ w444]
                        tunnel: w428 -> [_ w442]
                        tunnel: w427 -> [_ w438]
                        tunnel: w426 -> [_ w439]
                        frame False {
                          n168 = local write "error?"(w436) -> ()
                        }
                        frame True {
                          n169 = local read "Mode 4"() -> (w441:u16)
                          n170 = call "compliancevi3subvi.vi"("compliance (A)"=w443, "start"=w439, "compliance (V)"=w442, "total points"=w444, "step"=w438, "Mode"=w441) -> ("total points 2"=w440:u16, "compliance"=w437:dbl)  [unwired: 1 in, 1 out]
                          n171 = call "HP415xA _Config-Sweep-Secondary Sour.vi"("compliance"=w437, "step"=w438, "error in (no error)"=w447, "total points"=w440, "start"=w439, "VISA session"=w446) -> ("error out"=w445:errorcluster)  [unwired: 1 in]
                          n172 = local write "error?"(w445) -> ()
                        }
                      }
                    }
                    frame True {
                      n173 = local read "Mode 3"() -> (w458:u16)
                      n174 = call "compliancevi3subvi.vi"("compliance (A)"=w454, "start"=w450, "compliance (V)"=w452, "total points"=w453, "step"=w448, "Mode"=w458) -> ("total points 2"=w451:u16, "compliance"=w449:dbl)  [unwired: 1 in, 1 out]
                      n175 = call "HP415xA _Config-Sweep-Secondary Sour.vi"("compliance"=w449, "step"=w448, "error in (no error)"=w456, "total points"=w451, "start"=w450, "VISA session"=w457) -> ("error out"=w455:errorcluster)  [unwired: 1 in]
                      n176 = local write "error?"(w455) -> ()
                    }
                  }
                }
                frame True {
                  n177 = local read "Mode"() -> (w466:u16)
                  n178 = call "compliancevi3subvi.vi"("compliance (A)"=w464, "start"=w459, "compliance (V)"=w463, "total points"=w465, "step"=w461, "Mode"=w466) -> ("total points 2"=w460:u16, "compliance"=w462:dbl)  [unwired: 1 in, 1 out]
                  n179 = call "HP415xA _Config-Sweep-Secondary Sour.vi"("compliance"=w462, "step"=w461, "error in (no error)"=w468, "total points"=w460, "start"=w459, "VISA session"=w469) -> ("error out"=w467:errorcluster)  [unwired: 1 in]
                  n180 = local write "error?"(w467) -> ()
                }
              }
            }
          }
        }
        frame True {
          w478 = u16 2 items=["disabled", "Var1", "Var2", "Var1'", "Constant"] ("Function 2")
          n181 = local read "error?"() -> (w480:errorcluster)
          n182 = local read "Mode"() -> (w488:u16)
          n183 = local read "Function 2"() -> (w479:u16)
          n184 = call "compliancesubvi2.vi"("compliance (V)"=w487, "Mode"=w488, "compliance (A)"=w486) -> ("compliance"=w489:dbl)  [unwired: 3 in, 1 out]
          n185 = call "HP415xA _Config-Sweep-Primary Sour.vi"("step (linear only)"=w483, "stop"=w482, "start"=w481, "compliance"=w489, "error in (no error)"=w480, "sweep mode"=w484, "sweep spacing (linear: 0)"=w485, "VISA session"=w470) -> ("error out"=w471:errorcluster)  [unwired: 2 in]
          n186 = Equal?(x=w479, y=w478) -> (x = y?=w477:bool)
          n187 = case shown="True" w477 {
            tunnel: w476 -> [w495 w539]
            tunnel: w475 -> [w496 w538]
            tunnel: w474 -> [w493 w535]
            tunnel: w473 -> [w494 w537]
            tunnel: w472 -> [w492 w533]
            tunnel: w471 -> [w491 w542]
            tunnel: w470 -> [w490 w540]
            frame False {
              w499 = u16 2 items=["disabled", "Var1", "Var2", "Var1'", "Constant"] ("Function 2")
              n188 = local read "Function 3"() -> (w498:u16)
              n189 = Equal?(x=w498, y=w499) -> (x = y?=w497:bool)
              n190 = case shown="True" w497 {
                tunnel: w496 -> [w504 w522]
                tunnel: w495 -> [w505 w523]
                tunnel: w494 -> [w502 w528]
                tunnel: w493 -> [w503 w525]
                tunnel: w492 -> [w501 w524]
                tunnel: w491 -> [w506 w531]
                tunnel: w490 -> [w500 w529]
                frame False {
                  w509 = u16 2 items=["disabled", "Var1", "Var2", "Var1'", "Constant"] ("Function 2")
                  n191 = local read "Function 4"() -> (w508:u16)
                  n192 = Equal?(x=w508, y=w509) -> (x = y?=w507:bool)
                  n193 = case shown="True" w507 {
                    tunnel: w506 -> [w510 w521]
                    tunnel: w505 -> [_ w511]
                    tunnel: w504 -> [_ w512]
                    tunnel: w503 -> [_ w513]
                    tunnel: w502 -> [_ w518]
                    tunnel: w501 -> [_ w515]
                    tunnel: w500 -> [_ w519]
                    frame False {
                      n194 = local write "error?"(w510) -> ()
                    }
                    frame True {
                      n195 = local read "Mode 4"() -> (w517:u16)
                      n196 = call "compliancevi3subvi.vi"("compliance (A)"=w511, "start"=w513, "compliance (V)"=w512, "total points"=w518, "step"=w515, "Mode"=w517) -> ("total points 2"=w514:u16, "compliance"=w516:dbl)  [unwired: 1 in, 1 out]
                      n197 = call "HP415xA _Config-Sweep-Secondary Sour.vi"("compliance"=w516, "step"=w515, "error in (no error)"=w521, "total points"=w514, "start"=w513, "VISA session"=w519) -> ("error out"=w520:errorcluster)  [unwired: 1 in]
                      n198 = local write "error?"(w520) -> ()
                    }
                  }
                }
                frame True {
                  n199 = local read "Mode 3"() -> (w532:u16)
                  n200 = call "compliancevi3subvi.vi"("compliance (A)"=w523, "start"=w525, "compliance (V)"=w522, "total points"=w528, "step"=w524, "Mode"=w532) -> ("total points 2"=w527:u16, "compliance"=w526:dbl)  [unwired: 1 in, 1 out]
                  n201 = call "HP415xA _Config-Sweep-Secondary Sour.vi"("compliance"=w526, "step"=w524, "error in (no error)"=w531, "total points"=w527, "start"=w525, "VISA session"=w529) -> ("error out"=w530:errorcluster)  [unwired: 1 in]
                  n202 = local write "error?"(w530) -> ()
                }
              }
            }
            frame True {
              n203 = local read "Mode 2"() -> (w543:u16)
              n204 = call "compliancevi3subvi.vi"("compliance (A)"=w539, "start"=w535, "compliance (V)"=w538, "total points"=w537, "step"=w533, "Mode"=w543) -> ("total points 2"=w536:u16, "compliance"=w534:dbl)  [unwired: 1 in, 1 out]
              n205 = call "HP415xA _Config-Sweep-Secondary Sour.vi"("compliance"=w534, "step"=w533, "error in (no error)"=w542, "total points"=w536, "start"=w535, "VISA session"=w540) -> ("error out"=w541:errorcluster)  [unwired: 1 in]
              n206 = local write "error?"(w541) -> ()
            }
          }
        }
      }
    }
    frame #4 {
      # "This step sets the integration time."
      n207 = local read "VISA session"() -> (w544:refnum<visa-resource-name>)
      n208 = local read "error?"() -> (w548:errorcluster)
      n209 = call "HP415xA _Config-Meas-Timing.vi"("error in (no error)"=w548, "wait time parameter"="wait time parameter", "integration time"="integration time", "VISA session"=w544) -> ("error out"=w547:errorcluster)  [unwired: 2 in]
      n210 = local write "error?"(w547) -> ()
    }
    frame #5 {
      w584 = u32 1 items=["stop  ", "single  ", "single-append  ", "stress start  ", "continuous  ", "standby on  ", "standby off  ", "zero  "] ("function (stop:0)")
      w588 = u16 2 items=["disabled", "Var1", "Var2", "Var1'", "Constant"] ("Function")
      w593 = u16 1 items=["disabled", "Var1", "Var2", "Var1'", "Constant"] ("Function")
      n211 = local read "Function"() -> (w595:u16)
      n212 = local read "Function"() -> (w587:u16)
      n213 = Equal?(x=w595, y=w593) -> (x = y?=w594:bool)
      n214 = Equal?(x=w587, y=w588) -> (x = y?=w586:bool)
      n215 = case shown="False" w594 {
        tunnel: [w957 w972] -> w589
        tunnel: [w958 w971] -> _
        tunnel: w593 -> [w955 _]
        frame False {
          n216 = local read "Function 2"() -> (w959:u16)
          n217 = Equal?(x=w959, y=w955) -> (x = y?=w956:bool)
          n218 = case shown="False" w956 {
            tunnel: [w960 w970] -> w958
            tunnel: [w961 w969] -> w957
            tunnel: w955 -> [w964 _]
            frame False {
              n219 = local read "Function 3"() -> (w963:u16)
              n220 = Equal?(x=w963, y=w964) -> (x = y?=w962:bool)
              n221 = case shown="True" w962 {
                tunnel: [w966 w968] -> w961
                tunnel: [w965 w967] -> w960
                frame False {
                  n222 = local read "Vname 4"() -> (w966:string)
                  n223 = local read "Iname 4"() -> (w965:string)
                }
                frame True {
                  n224 = local read "Vname 3"() -> (w968:string)
                  n225 = local read "Iname 3"() -> (w967:string)
                }
              }
            }
            frame True {
              n226 = local read "Vname 2"() -> (w969:string)
              n227 = local read "Iname 2"() -> (w970:string)
            }
          }
        }
        frame True {
          n228 = local read "Vname"() -> (w972:string)
          n229 = local read "Iname"() -> (w971:string)
        }
      }
      n230 = case shown="False" w586 {
        tunnel: [w899 w952] -> w559
        tunnel: [w898 TRUE ("x = y?")] -> w565
        frame False {
          w902 = u16 2 items=["disabled", "Var1", "Var2", "Var1'", "Constant"] ("Function")
          n231 = local read "Function 2"() -> (w901:u16)
          n232 = Equal?(x=w901, y=w902) -> (x = y?=w900:bool)
          n233 = case shown="False" w900 {
            tunnel: [w904 w942] -> w899
            tunnel: [w903 TRUE ("x = y?")] -> w898
            frame False {
              w907 = u16 2 items=["disabled", "Var1", "Var2", "Var1'", "Constant"] ("Function")
              n234 = local read "Function 3"() -> (w906:u16)
              n235 = Equal?(x=w906, y=w907) -> (x = y?=w905:bool)
              n236 = case shown="False" w905 {
                tunnel: [w912 w932] -> w904
                tunnel: [w908 TRUE ("x = y?")] -> w903
                frame False {
                  w911 = u16 2 items=["disabled", "Var1", "Var2", "Var1'", "Constant"] ("Function")
                  n237 = local read "Function 4"() -> (w910:u16)
                  n238 = Equal?(x=w910, y=w911) -> (x = y?=w909:bool)
                  n239 = case shown="False" w909 {
                    tunnel: ["0" ("Vname 4") w922] -> w912
                    tunnel: [FALSE ("x = y?") TRUE ("x = y?")] -> w908
                    frame False {
                    }
                    frame True {
                      w916 = u16 2 items=["V", "I", "VPulse", "IPulse", "Common"] ("Mode 2")
                      w919 = u16 0 items=["V", "I", "VPulse", "IPulse", "Common"] ("Mode 2")
                      n240 = local read "Mode 4"() -> (w918:u16)
                      n241 = Equal?(x=w919, y=w918) -> (x = y?=w920:bool)
                      n242 = Equal?(x=w918, y=w916) -> (x = y?=w917:bool)
                      n243 = Or(x=w920, y=w917) -> (x .or. y?=w915:bool)
                      n244 = case shown="False" w915 {
                        tunnel: [w923 w924] -> w922
                        frame False {
                          n245 = local read "Iname 4"() -> (w923:string)
                        }
                        frame True {
                          n246 = local read "Vname 4"() -> (w924:string)
                        }
                      }
                    }
                  }
                }
                frame True {
                  w928 = u16 2 items=["V", "I", "VPulse", "IPulse", "Common"] ("Mode 2")
                  w927 = u16 0 items=["V", "I", "VPulse", "IPulse", "Common"] ("Mode 2")
                  n247 = local read "Mode 3"() -> (w926:u16)
                  n248 = Equal?(x=w927, y=w926) -> (x = y?=w930:bool)
                  n249 = Equal?(x=w926, y=w928) -> (x = y?=w929:bool)
                  n250 = Or(x=w930, y=w929) -> (x .or. y?=w925:bool)
                  n251 = case shown="False" w925 {
                    tunnel: [w933 w934] -> w932
                    frame False {
                      n252 = local read "Iname 3"() -> (w933:string)
                    }
                    frame True {
                      n253 = local read "Vname 3"() -> (w934:string)
                    }
                  }
                }
              }
            }
            frame True {
              w936 = u16 2 items=["V", "I", "VPulse", "IPulse", "Common"] ("Mode 2")
              w937 = u16 0 items=["V", "I", "VPulse", "IPulse", "Common"] ("Mode 2")
              n254 = local read "Mode 2"() -> (w938:u16)
              n255 = Equal?(x=w937, y=w938) -> (x = y?=w940:bool)
              n256 = Equal?(x=w938, y=w936) -> (x = y?=w939:bool)
              n257 = Or(x=w940, y=w939) -> (x .or. y?=w935:bool)
              n258 = case shown="True" w935 {
                tunnel: [w943 w944] -> w942
                frame False {
                  n259 = local read "Iname 2"() -> (w943:string)
                }
                frame True {
                  n260 = local read "Vname 2"() -> (w944:string)
                }
              }
            }
          }
        }
        frame True {
          w949 = u16 2 items=["V", "I", "VPulse", "IPulse", "Common"] ("Mode")
          w950 = u16 0 items=["V", "I", "VPulse", "IPulse", "Common"] ("Mode")
          n261 = local read "Mode"() -> (w948:u16)
          n262 = Equal?(x=w948, y=w950) -> (x = y?=w947:bool)
          n263 = Equal?(x=w948, y=w949) -> (x = y?=w946:bool)
          n264 = Or(x=w947, y=w946) -> (x .or. y?=w945:bool)
          n265 = case shown="True" w945 {
            tunnel: [w953 w954] -> w952
            frame False {
              n266 = local read "Iname"() -> (w953:string)
            }
            frame True {
              n267 = local read "Vname"() -> (w954:string)
            }
          }
        }
      }
      n268 = local read "error?"() -> (w576:errorcluster)
      n269 = Unbundle("Y2 axis settings") -> ("Y2 axis on/off"=w568:bool, "MINIMUM"=w581:ext, "MAXIMUM"=w580:ext, "Variable name"=w572:string, "LIN or LOG axis"=w579:string)
      n270 = local read "Var2 step settings"() -> (w591:T3)
      n271 = local read "Var1 sweep settings"() -> (w592:T4)
      n272 = local read "VISA session"() -> (w560:refnum<visa-resource-name>)
      n273 = call "Y1subvi.vi"("MAXIMUM"="MAXIMUM", "Variable name"="Y1 axis", "error in (no error)"=w576, "MINIMUM"="MINIMUM", "LIN or LOG axis"="LIN", "VISA resource name"=w560) -> ("error out"=w577:errorcluster)
      n274 = case shown="False" w568 {
        tunnel: w577 -> [w890 w897]
        tunnel: w560 -> [_ w896]
        tunnel: w581 -> [_ w895]
        tunnel: w580 -> [_ w894]
        tunnel: w572 -> [_ w893]
        tunnel: w579 -> [_ w892]
        tunnel: [w890 w891] -> w578
        frame False {
        }
        frame True {
          n275 = call "Y2subvi.vi"("MAXIMUM"=w894, "Variable name"=w893, "error in (no error)"=w897, "MINIMUM"=w895, "LIN or LOG axis"=w892, "VISA resource name"=w896) -> ("error out"=w891:errorcluster)
        }
      }
      n276 = Unbundle(w591) -> ("total points"=w590:u16)  [unwired: 4 out]
      n277 = Decrement(x=w590) -> (x-1=w550:u16)
      n278 = Unbundle(w592) -> ("start"=w558:dbl)  [unwired: 6 out]
      n279 = call "HP415xA Op-Start-Stop.vi"("error in (no error)"=w578, "function (stop:0)"=w584, "wait until finish"=TRUE, "VISA session"=w560) -> ("error out"=w583:errorcluster)  [unwired: 6 in, 1 out]
      n280 = call "HP415xA Op-Download Trace.vi"("error in (no error)"=w583, "trace (variable) name"=w589, "VISA session"=w560) -> ("error out"=w598:errorcluster, "trace"=w566:dbl[])
      n281 = call "HP415xA Op-Download Trace.vi"("error in (no error)"=w598, "trace (variable) name"="Y1 axis", "VISA session"=w560) -> ("error out"=w573:errorcluster, "trace"=w561:dbl[])
      n282 = case shown="False" w568 {
        tunnel: w573 -> [w875 w883]
        tunnel: w560 -> [_ w882]
        tunnel: w572 -> [_ w881]
        tunnel: [w875 w880] -> w562
        tunnel: w566 -> [w873 w879]
        tunnel: w561 -> [w874 w878]
        tunnel: [w872 w877] -> w569
        tunnel: [dbl[] [] ("trace") w876] -> w567
        frame False {
          n283 = Bundle("trace"=w873, "trace"=w874) -> (w872:cluster{"trace":dbl[], "trace":dbl[]})  [unwired: 1 in]
        }
        frame True {
          n284 = call "HP415xA Op-Download Trace.vi"("error in (no error)"=w883, "trace (variable) name"=w881, "VISA session"=w882) -> ("error out"=w880:errorcluster, "trace"=w876:dbl[])
          n285 = stacked-sequence {
            tunnel: w876 -> [_ w888]
            tunnel: w879 -> [w886 w887]
            tunnel: w878 -> [w885 _]
            tunnel: [w884 _] -> w877
            frame #0 {
              n286 = Bundle("trace"=w886, "trace"=w885) -> (w884:cluster{"trace":dbl[], "trace":dbl[]})  [unwired: 1 in]
            }
            frame #1 {
              n287 = Bundle("trace"=w887, "trace"=w888) -> (→"graphic display 2":cluster{"trace":dbl[], "trace":dbl[]})  [unwired: 1 in]
            }
          }
        }
      }
      "graphic display" <- w569
      n288 = case shown="True" w565 {
        tunnel: w558 -> [_ w743]
        tunnel: w561 -> [w603 w742]
        tunnel: w566 -> [w604 w740]
        tunnel: w550 -> [_ w739]
        tunnel: w560 -> [_ w735]
        tunnel: w562 -> [_ w734]
        tunnel: [w605 w733] -> w564
        tunnel: w559 -> [_ w732]
        tunnel: w559 -> [_ w725]
        tunnel: [dbl[] [] ("trace") w731] -> w563
        tunnel: w557 -> [_ w728]
        tunnel: w556 -> [_ w727]
        tunnel: w555 -> [_ w676]
        tunnel: [_ w652] -> w554
        tunnel: [_ w654] -> w553
        tunnel: w552 -> [_ w693]
        tunnel: w551 -> [_ w692]
        tunnel: w550 -> [_ _]
        tunnel: w549 -> [_ w687]
        frame False {
          n289 = Build Array(w604, w603) -> (w600:dbl[][])
          n290 = local read "error? 2"() -> (w605:errorcluster)
          n291 = call-poly <vilib>:"Write To Spreadsheet File.vi"("transpose? (no:F)"=TRUE ("append to file? (new file:F)"), "format (%.3f)"="%.5e", "2D data"=w600) -> ()  [unwired: 5 in, 1 out]
        }
        frame True {
          w646 = 2
          w647 = 2
          w660 = 0
          w658 = 0
          (unwired) 0.000115
          w717 = "%s"
          w667 = "\r"
          n292 = Initialize Array("") -> (w706:string[])  [unwired: 1 in]
          n293 = call "HP415xA Op-Download Trace.vi"("error in (no error)"=w734, "trace (variable) name"=w732, "VISA session"=w735) -> ("error out"=w733:errorcluster, "trace"=w731:dbl[])
          n294 = for {
            N: w739 -> [w798]
            shift-right: [w815] -> w652
            shift-left: w740 -> [w811]
            tunnel: w743 -> [w817]
            tunnel: [w816] -> _ mode=indexing
            shift-right: [w812] -> w654
            shift-left: w742 -> [w814]
            tunnel: [w813] -> w741 mode=indexing
            shift-right: [w808] -> w721
            shift-left: w731 -> [w810]
            tunnel: w725 -> [_]
            tunnel: [w802] -> w723 mode=indexing
            shift-right: [w801] -> w710
            shift-left: w706 -> [w800]
            tunnel: [w798] -> _ mode=indexing
            n295 = Search 1D Array(1D array=w811, element=w817, start index (0)=1) -> (index of element=w809:i32)
            n296 = Split 1D Array(array=w810, index=w809) -> (first subarray=w806:dbl[], second subarray=w808:dbl[])
            n297 = Array Size(array=w806) -> (size(s)=w805:i32)
            n298 = Decrement(x=w805) -> (x-1=w804:i32)
            n299 = Split 1D Array(array=w814, index=w809) -> (first subarray=w813:dbl[], second subarray=w812:dbl[])
            n300 = Split 1D Array(array=w811, index=w809) -> (first subarray=w816:dbl[], second subarray=w815:dbl[])
            n301 = Array Subset(array=w806, index=w804) -> (w807:dbl[])  [unwired: 1 in]
            n302 = Number To Exponential String(number=w807) -> (E-format string=w803:string[])  [unwired: 3 in]
            n303 = Concatenate Strings(w803) -> (w802:string)
            n304 = Build Array (concatenate)("Id", w800) -> (w801:string[])
          }
          n305 = Build Array (concatenate)(w652, w741, w654) -> (w738:dbl[][])
          n306 = Transpose 2D Array(2D array=w738) -> (transposed array=w736:dbl[][])
          n307 = Array To Spreadsheet String(array=w736, 3:"%.5e" ("format string")) -> (spreadsheet string=w726:string)  [unwired: 1 in]
          n308 = local read "Temp (K)"() -> (w643:dbl)
          n309 = Number To Exponential String(number=w643) -> (E-format string=w642:string)  [unwired: 3 in]
          n310 = Build Array("Sample Temp (K):", w642) -> (w641:string[])
          n311 = Build Array("Vg", "Id") -> (w711:string[])
          n312 = Array Size(array=w721) -> (size(s)=w722:i32)
          n313 = Reshape Array(w641, 1 ("start index (0)")) -> (w638:string[])
          n314 = Decrement(x=w722) -> (x-1=w720:i32)
          n315 = Array Subset(array=w721, index=w720) -> (w719:dbl[])  [unwired: 1 in]
          n316 = Insert Into Array(array=w711, index=2, new element=w710) -> (w709:string[])
          n317 = Number To Exponential String(number=w719) -> (E-format string=w715:string[])  [unwired: 3 in]
          n318 = Array To Spreadsheet String(array=w638, 3:"%s") -> (spreadsheet string=w637:string)  [unwired: 1 in]
          n319 = Array To Spreadsheet String(array=w709, 3:w717) -> (spreadsheet string=w716:string)  [unwired: 1 in]
          n320 = Concatenate Strings(w715) -> (w714:string)
          n321 = Build Array (concatenate)("Vd=", w723, w714) -> (w718:string[])
          n322 = Array To Spreadsheet String(array=w718, 3:w717) -> (spreadsheet string=w724:string)  [unwired: 1 in]
          n323 = Fract/Exp String To Number(string="") -> (number=w626:dbl)  [unwired: 3 in, 1 out]
          n324 = local read "Vt"() -> (w636:dbl)
          n325 = Build Array("Mobility-Sat (cm^2/Vs):", "Mobility-Lin (cm^2/Vs):", "On/Off I-Sat:", "Off I-Sat (A):", "Vt-Sat (V):", "STS-Sat (V/decade):", "Trap Density-VT (Traps/Vcm^2):", "Trap Density-STS (Traps/Vcm^2):") -> (w674:string[])
          n326 = Array Size(array=w652) -> (size(s)=w680:i32)
          n327 = Subtract(x=w680, y="NumPts") -> (x-y=w691:dbl)
          n328 = Initialize Array(0) -> (w690:i32[])  [unwired: 1 in]
          n329 = Initialize Array(w658, w647) -> (w659:i32[])
          n330 = Initialize Array(w658, w647) -> (w657:i32[])
          n331 = Initialize Array(w658) -> (w662:i32[])  [unwired: 1 in]
          n332 = for {
            N: w680 -> [w746]
            shift-right: [w749] -> w679
            shift-left: w654 -> [w750]
            i -> [w745]
            n333 = Subtract(x=w746, y=w745) -> (x-y=w744:i32)
            n334 = Index Array(array=w750, index=w744) -> (element=w747:dbl)
            n335 = Greater Or Equal To 0?(x=w747) -> (x >= 0?=w748:bool)
            n336 = case shown="False" w748 {
              tunnel: w750 -> [w751 w754]
              tunnel: w744 -> [_ w752]
              tunnel: [w751 w753] -> w749
              frame False {
              }
              frame True {
                n337 = Delete From Array(array=w754, index=w752) -> (array with subset deleted=w753:dbl[])  [unwired: 1 in, 1 out]
              }
            }
          }
          n338 = for {
            N: w691 -> [_]
            shift-right: [w792] -> _
            shift-left: w652 -> [w792]
            shift-right: [w793] -> _
            shift-left: w654 -> [w793]
            shift-right: [w797] -> w696
            shift-left: w690 -> [w796]
            shift-right: [w795] -> w694
            shift-left: w662 -> [w794]
            tunnel: "NumPts" -> [w787]
            shift-right: [w783] -> w661
            shift-left: w659 -> [w786]
            shift-right: [w780] -> w650
            shift-left: w657 -> [w781]
            i -> [w784]
            n339 = Array Subset(array=w792, index=w784, length=w787) -> (w782:dbl[])
            n340 = Array Subset(array=w793, index=w784, length=w787) -> (w791:dbl[])
            n341 = Absolute Value(x=w791) -> (abs(x)=w790:dbl[])
            n342 = Build Array (concatenate)(w781, w782) -> (w780:dbl[])
            n343 = Square Root(x=w790) -> (sqrt(x)=w785:dbl[])
            n344 = call <vilib>:"Linear Fit.vi"("Y"=w785, "X"=w782) -> ("Best Linear Fit"=w789:dbl[], "slope"=w779:dbl, "intercept"=w777:dbl)  [unwired: 9 in, 2 out]
            n345 = Insert Into Array(array=w786, index=w784, new element=w785) -> (w783:i32[])
            n346 = call <vilib>:"Goodness of Fit.vi"("Best Fit"=w789, "Y"=w785) -> ("R-square"=w788:dbl)  [unwired: 6 in, 3 out]
            n347 = Negate(x=w779) -> (-x=w778:dbl)
            n348 = Divide(x=w778, y=w777) -> ()  [unwired: 1 out]
            n349 = Build Array (concatenate)(w794, w788) -> (w795:dbl[])
            n350 = Build Array (concatenate)(w796, w779) -> (w797:dbl[])
          }
          n351 = Absolute Value(x=w654) -> (abs(x)=w656:dbl[])
          n352 = Array Max & Min(array=w679) -> (max value=w677:dbl, min value=w678:dbl)  [unwired: 2 out]
          n353 = Square Root(x=w656) -> (sqrt(x)=w655:dbl[])
          n354 = Initialize Array(w660, w646) -> (w649:i32[])
          n355 = Initialize Array(w660, w646) -> (w666:i32[])
          n356 = Divide(x=w678, y=w677) -> (x/y=w628:dbl)
          n357 = for {
            N: 20 -> [_]
            shift-right: [w775] -> _
            shift-left: w694 -> [w776]
            shift-right: [w767] -> _
            shift-left: w696 -> [w765]
            shift-right: [w766] -> w697
            shift-left: w666 -> [w774]
            shift-right: [w773] -> w688
            shift-left: w666 -> [w772]
            shift-right: [w763] -> _
            shift-left: w661 -> [w764]
            shift-right: [w762] -> w615
            shift-left: w649 -> [w770]
            shift-right: [w755] -> _
            shift-left: w650 -> [w757]
            shift-right: [w759] -> w614
            shift-left: w649 -> [w758]
            w761 = 1
            n358 = Array Max & Min(array=w776) -> (max value=w771:dbl, max index (indices)=w756:i32)  [unwired: 2 out]
            n359 = Array Subset(array=w757, index=w756, length=w761) -> (w760:dbl[])
            n360 = Array Subset(array=w764, index=w756, length=w761) -> (w769:i32[])
            n361 = Array Subset(array=w765, index=w756, length=w761) -> (w768:dbl[])
            n362 = Build Array (concatenate)(w774, w768) -> (w766:dbl[])
            n363 = Delete From Array(array=w776, index=w756) -> (array with subset deleted=w775:dbl[])  [unwired: 1 in, 1 out]
            n364 = Build Array (concatenate)(w758, w760) -> (w759:dbl[])
            n365 = Build Array (concatenate)(w772, w771) -> (w773:dbl[])
            n366 = Build Array (concatenate)(w770, w769) -> (w762:i32[])
            n367 = Delete From Array(array=w764, index=w756) -> (array with subset deleted=w763:i32[])  [unwired: 1 in, 1 out]
            n368 = Delete From Array(array=w757, index=w756) -> (array with subset deleted=w755:dbl[])  [unwired: 1 in, 1 out]
            n369 = Delete From Array(array=w765, index=w756) -> (array with subset deleted=w767:dbl[])  [unwired: 1 in, 1 out]
          }
          "Max R" <- w688
          n370 = local write "On/Off Current"(w628) -> ()
          n371 = Bundle("trace"=w652, w655) -> (w653:cluster{"trace":dbl[], dbl[]})  [unwired: 1 in]
          n372 = Fract/Exp String To Number(string=w693) -> (number=w664:dbl)  [unwired: 3 in, 1 out]
          n373 = local read "Vt"() -> (w635:dbl)
          n374 = Fract/Exp String To Number(string=w692) -> (number=w665:dbl)  [unwired: 3 in, 1 out]
          n375 = Fract/Exp String To Number(string=w687) -> (number=w682:dbl)  [unwired: 3 in, 1 out]
          n376 = Array Max & Min(array=w697) -> (min value=w648:dbl, min index (indices)=w617:i32)  [unwired: 2 out]
          n377 = Multiply(x=w617, y="NumPts") -> (x*y=w619:dbl)
          n378 = Array Subset(array=w614, index=w619, length="NumPts") -> (w620:dbl[])
          n379 = Array Subset(array=w615, index=w619, length="NumPts") -> (w621:i32[])
          n380 = call <vilib>:"Linear Fit.vi"("Y"=w621, "X"=w620) -> ("slope"=w624:dbl, "intercept"=w622:dbl)  [unwired: 9 in, 3 out]
          n381 = Negate(x=w622) -> (-x=w623:dbl)
          n382 = Divide(x=w623, y=w624) -> (x/y=w618:dbl)
          n383 = Bundle(w620, w621) -> (w613:cluster{dbl[], i32[]})  [unwired: 1 in]
          n384 = local write "Vt"(w618) -> ()
          n385 = Build Array(w653, w613) -> (→"XY Graph":cluster{"trace":dbl[], dbl[]}[])
          n386 = Absolute Value(x=w635) -> (abs(x)=w634:dbl)
          n387 = Square(x=w648) -> (x^2=w698:dbl)
          n388 = Multiply(x=2, y=w698) -> (x*y=w699:dbl)
          n389 = Multiply(x=3.9, y=8.854e-12) -> (x*y=w684:dbl)
          n390 = Multiply(x=w665, y=w699) -> (x*y=w700:dbl)
          n391 = Multiply(x=w682, y=1e-09) -> (x*y=w681:dbl)
          n392 = Divide(x=w684, y=w681) -> (x/y=w633:dbl)
          n393 = Multiply(x=w634, y=w633) -> (x*y=w632:dbl)
          n394 = Divide(x=w632, y=1.602e-19) -> (x/y=w629:dbl)
          n395 = Multiply(x=w664, y=w633) -> (x*y=w701:dbl)
          n396 = Divide(x=w700, y=w701) -> (x/y=w703:dbl)
          n397 = Multiply(x=w703, y=10000) -> (x*y=w630:dbl)
          n398 = Build Array(w630, w628, w636, w626, w629, w626) -> (w673:dbl[])
          n399 = Number To Exponential String(number=w673) -> (E-format string=w672:string[])  [unwired: 3 in]
          n400 = Build Array(w674, w672) -> (w671:string[][])
          n401 = Transpose 2D Array(2D array=w671) -> (transposed array=w670:string[][])
          n402 = Array To Spreadsheet String(array=w670, 3:"%s") -> (spreadsheet string=w668:string)  [unwired: 1 in]
          n403 = Concatenate Strings(w728, w667, w727, w667, w676, w637, w667, w668, w667, w724, w716, w726, "\r") -> (w730:string)
          n404 = call <vilib>:"Write Characters To File.vi"("append to file? (new file:F)"=TRUE, "character string"=w730, "file path (dialog if empty)"="Input Path") -> ("new file path (Not A Path if cancelled)"=w625:path)  [unwired: 2 in]
          n405 = local write "Output Path"(w625) -> ()
          n406 = local write "Trap Density-VT"(w629) -> ()
          n407 = local write "Mobility"(w630) -> ()
        }
      }
      n408 = case shown="True" w568 {
        tunnel: w550 -> [_ w824]
        tunnel: w565 -> [_ w825]
        tunnel: w566 -> [_ w823]
        tunnel: w558 -> [_ w822]
        tunnel: w567 -> [_ w821]
        tunnel: w563 -> [_ w820]
        tunnel: w559 -> [_ w819]
        frame False {
        }
        frame True {
          n409 = case shown="True" w825 {
            tunnel: w824 -> [_ w841]
            tunnel: w823 -> [w829 w856]
            tunnel: w822 -> [_ w855]
            tunnel: w821 -> [w830 w854]
            tunnel: w820 -> [_ w853]
            tunnel: w819 -> [_ w836]
            frame False {
              n410 = Build Array(w829, w830) -> (w828:dbl[][])
              n411 = call-poly <vilib>:"Write To Spreadsheet File.vi"("transpose? (no:F)"=TRUE, "format (%.3f)"="%.5e", "2D data"=w828) -> ()  [unwired: 5 in, 1 out]
            }
            frame True {
              n412 = for {
                N: w841 -> [_]
                shift-right: [w867] -> w852
                shift-left: w856 -> [w868]
                tunnel: w855 -> [w870]
                tunnel: [w866] -> _ mode=indexing
                shift-right: [w863] -> w850
                shift-left: w854 -> [w865]
                tunnel: [w864] -> w851 mode=indexing
                shift-right: [w860] -> w845
                shift-left: w853 -> [w861]
                tunnel: [w857] -> w842 mode=indexing
                n413 = Search 1D Array(1D array=w868, element=w870, start index (0)=1) -> (index of element=w862:i32)
                n414 = Split 1D Array(array=w868, index=w862) -> (first subarray=w866:dbl[], second subarray=w867:dbl[])
                n415 = Split 1D Array(array=w865, index=w862) -> (first subarray=w864:dbl[], second subarray=w863:dbl[])
                n416 = Split 1D Array(array=w861, index=w862) -> (first subarray=w858:dbl[], second subarray=w860:dbl[])
                n417 = Index Array(array=w858, index=1) -> (element=w857:dbl)
              }
              n418 = Build Array (concatenate)(w852, w851, w850) -> (w849:dbl[][])
              n419 = Index Array(array=w845, index=1) -> (element=w843:dbl)
              n420 = Transpose 2D Array(2D array=w849) -> (transposed array=w848:dbl[][])
              n421 = Insert Into Array(array=w842, index=w841, new element=w843) -> (w840:dbl[])
              n422 = Array To Spreadsheet String(delimiter (Tab)=",", array=w840, 3:"%.5e" ("format string")) -> (spreadsheet string=w834:string)
              n423 = Array To Spreadsheet String(delimiter (Tab)=",", array=w848, 3:"%.5e" ("format string")) -> (spreadsheet string=w832:string)
              n424 = Concatenate Strings(w836, "," ("string")) -> (w835:string)
              n425 = Concatenate Strings(w835, w834) -> (w833:string)
              n426 = Concatenate Strings(w833, w832) -> (w831:string)
              n427 = call <vilib>:"Write Characters To File.vi"("character string"=w831) -> ()  [unwired: 4 in, 1 out]
            }
          }
        }
      }
      n428 = call "HP415xA Sys-Error Query.vi"("VISA session"=w560, "error in (no error)"=w564) -> ("error out"=w596:errorcluster)  [unwired: 2 in, 1 out]
      n429 = call "HP415xA  Close.vi"("error in (no error)"=w596, "VISA session"=w560) -> ("error out"=w597:errorcluster)
      n430 = local write "error?"(w597) -> ()
    }
    frame #6 {
      n431 = flat-sequence {
        frame #0 {
          n432 = local read "Output Path"() -> (w987:path)
          n433 = local read "Sample Properties:"() -> (w983:T1)
          n434 = local read "Temp (K)"() -> (w974:dbl)
          n435 = call "sub_thresh_swing_subvi.vi"("Path"=w987) -> ("Sub Threshold Swing"=w973:dbl)  [unwired: 10 in, 4 out]
          n436 = Unbundle By Name(w983) -> ("SiO2 Thickness"=w976:string)
          n437 = Equal To 0?(x=w974) -> (x = 0?=w986:bool)
          n438 = local write "STS"(w973) -> ()
          n439 = case shown="True" w986 {
            tunnel: [w988 290] -> w985
            tunnel: w974 -> [w988 _]
            frame False {
            }
            frame True {
            }
          }
          n440 = Fract/Exp String To Number(string=w976) -> (number=w978:dbl)  [unwired: 3 in, 1 out]
          n441 = Multiply(x=3.9, y=8.854e-12) -> (x*y=w982:dbl)
          n442 = Multiply(x=w978, y=1e-09) -> (x*y=w979:dbl)
          n443 = Divide(x=w982, y=w979) -> (x/y=w975:dbl)
          n444 = call "Trap Density_STS.vi"("Temp (T) [K]"=w985, "S.T.S. (S)"=w973, "Dielectric"=w975) -> ("Trap Density (N)"=w984:dbl)  [unwired: 8 in]
          n445 = local write "Trap Density-STS"(w984) -> ()
        }
        frame #1 {
          n446 = local read "Output Path"() -> (w990:path)
          n447 = call-poly <vilib>:"Read From Spreadsheet File.vi"("file path (dialog if empty)"=w990) -> ("all rows"=w997:string[][])  [unwired: 6 in, 4 out]
          n448 = Array Subset(array=w997, index (col)=0, length (col)=1) -> (w1005:string[][])  [unwired: 2 in]
          n449 = Reshape Array(w1005, 100) -> (w1002:string[])
          n450 = Search 1D Array(1D array=w1002, element="S.T.S. (V/decade):") -> (index of element=w1000:i32)  [unwired: 1 in]
          n451 = Search 1D Array(1D array=w1002, element="Trap Density-STS (Traps/Vcm^2):") -> (index of element=w994:i32)  [unwired: 1 in]
          n452 = local read "Trap Density-STS"() -> (w993:dbl)
          n453 = local read "STS"() -> (w1001:dbl)
          n454 = Number To Exponential String(number=w1001) -> (E-format string=w998:string)  [unwired: 3 in]
          n455 = Replace Array Subset(array=w997, new element=w998, index (row)=w1000, index (col)=1) -> (w996:string[][])
          n456 = Number To Exponential String(number=w993) -> (E-format string=w992:string)  [unwired: 3 in]
          n457 = Replace Array Subset(array=w996, new element=w992, index (row)=w994, index (col)=1) -> (w991:string[][])
          "Array" <- w991
          n458 = call-poly <vilib>:"Write To Spreadsheet File.vi"("2D data"=w991, "file path (dialog if empty)"=w990) -> ()  [unwired: 6 in, 1 out]
        }
      }
    }
  }
